vi "Control Experiment SM.vi"() -> ()   [LabVIEW 2016, in "Control Experiment SM.lvclass"]
doc: "Use this VI to help configure your experiment.\n1. Choose Pickering or Not Pickering\n2. Configure the Electrode control to show which electrode is connected to which lockin\n3. Choose a Label for each electrode to configure Krohn Hite amplifier automatically\n4. Easily set all Krohn Hite channels to be \"all ground\" or \"all differential\" mode\n5. Fill out information about you and your device in the lower left corner\n6. When you are finished, or when you want to update the amplifiers, click the \"CREATE OUTPUT\" button located in upper right. Clicking this button will set the amplifiers, Pickering switch (if you have one), and write information to a functional global variable that you can easily read from elsewhere in your program"
uses:
  Control Experiment SM.lvclass
  <vilib>/addons/_JKI.lib/Serialization/JSON/JKI JSON Serialization.lvlib
  Typedefs/KH Mode-enum.ctl
  <userlib>/LevyLab/Krohn Hite 7008/typedefs/Gain-Enum.ctl
  <userlib>/LevyLab/Krohn Hite 7008/Instrument.KH7008.lvclass
  <userlib>/LevyLab/Krohn Hite 7008/typedefs/Shunt-Enum.ctl
  <userlib>/LevyLab/Krohn Hite 7008/typedefs/Input Configuration-Enum.ctl
  <userlib>/_MGI/File/MGI Create Directory Chain Behavior Enum.ctl
  <vilib>/addons/_JKI.lib/REST Client/classes/REST Client/HTTP Header.ctl
  <vilib>/addons/_JKI.lib/REST Client/classes/REST Client/REST Client.lvclass
  <vilib>/JKI/JKI SMO/SMO/SMO.lvclass
  <userlib>/LevyLab/Lockin-Multichannel/Instrument.Lockin/Instrument.Lockin.lvclass
  Typedefs/Control Experiment JSON--cluster.ctl
  <vilib>/Utility/sysdir.llb/System Directory Type.ctl
  <userlib>/LevyLab/Levylab Instruments/SMOs/Configuration/Configuration.lvclass
  Typedefs/Instrument--enum.ctl
  Typedefs/UI Controls --cluster.ctl
  <userlib>/_OpenG.lib/array/array.llb/Remove Duplicates from 1D Array (Variant)__ogtk.vi
  <userlib>/LevyLab/Krohn Hite 7008/typedefs/Channel-Enum.ctl
  <userlib>/LevyLab/Krohn Hite 7008/typedefs/Filter-Enum.ctl
  <userlib>/LevyLab/Krohn Hite 7008/typedefs/Coupling-Enum.ctl
  <userlib>/LevyLab/Krohn Hite 7008/typedefs/SetAll-Cluster.ctl
  <userlib>/LevyLab/Krohn Hite 7008/typedefs/SetAll-Array.ctl
  <userlib>/LevyLab/Levylab Instruments/SMOs/Logger.PGSQL/Logger.PGSQL.lvclass
  <userlib>/_OpenG.lib/file/file.llb/File Exists - Scalar__ogtk.vi
  <vilib>/Platform/browser.llb/Open URL in Default Browser (string).vi
  <userlib>/LevyLab/Levylab Instruments/Instrument Types/CBridge/Instrument.CBridge.lvclass
  <userlib>/LevyLab/Levylab Instruments/Instrument Types/Strain/Instrument.Strain.lvclass
  C:/Program Files (x86)/National Instruments/LabVIEW 2016/vi.lib/JKI/JKI SMO/SMO/SMO.lvclass
  <userlib>/LevyLab/Levylab Instruments/Instrument Types/Cryostat/Instrument.Cryostat.lvclass
  <userlib>/LevyLab/Levylab Instruments/Instrument Types/Optical Delay Line/Instrument.OpticalDelayLine.lvclass
  <userlib>/LevyLab/Levylab Instruments/Instrument Types/VNA/Instrument.VNA.lvclass
  <userlib>/LevyLab/Levylab Instruments/Instrument Types/VSource/Instrument.VSource.lvclass
panel:
  in  "I'm Finished Taking Data!":bool
  out "Values have changed":bool
  in  "Create Output":bool
  in  "OK":bool
  out "Control Experiment":refnum<class "Control Experiment SM.lvclass">
  in  "C.E.":refnum<class "Control Experiment SM.lvclass">
  in  "Tab Control":T1(tab)
  in  "DC Coupled":bool=TRUE
  in  "Bandwidth Filter":bool=TRUE
  in  "#AO":u32=8
  in  "Gain":dbl[](array[numeric])=[1.0, 1.0, 1.0, 1.0, 1.0, 1.0, 1.0, 1.0]
  in  "KH":T5={"KH #"=[0, 1, 2, 3, 4, 5, 6, 7], "KH Configuration"=[enum."Differential", enum."Differential", enum."SE+ (-gnd)", enum."SE+ (-gnd)", enum."Ground", enum."Differential", enum."Ground", enum."Differential"], "KH Gain"=[enum."1x", enum."1000x", enum."1x", enum."10x", enum."1x", enum."1x", enum."1x", enum."1x"], "KH Shunt Resistor"=[enum."50k Ohms", enum."50k Ohms", enum."Open", enum."Open", enum."Open", enum."50k Ohms", enum."Open", enum."Open"]}
  in  "Lockin":T7={"AI"=[1, 2, 3, 4, 5, 6, 7, 8], "Electrode"=["1", "2", "4", "3", "", "26", "", ""], "Label"=[2, 14, 3, 4, 0, 1, 0, 0], "Electrode Config"=[enum."Current", enum."Gate", enum."Voltage (SE)", enum."Voltage (SE)", enum."Ground", enum."Current", enum."Ground", enum."Voltage (Diff)"]} {"Label" items=["", "I+", "I-", "V1+", "V1-", "V2+", "V2-", "V3+", "V3-", "V4+", "V4-", "dV1", "dV2", "dV3", "Vsg", "Vbg"]}
  in  "#AI":u32=8
  in  "KH All Buttons":T8(radio)
  in  "Defualt Shunt Resistor":T4=enum."50k Ohms"
  in  "Description":string="this is a test"
  in  "Sample (SAXXXX)":string="TEST"
  in  "Device (YYYYMMDD)":string="20200113"
  in  "Instrument":T9
  in  "Username":string="Patrick"
  in  "non KH":T10={"AO"=[], "Electrodes 2"=["27"], "Labels 2"=[1], "unused"=[]} {"Labels 2" items=["", "I+", "I-", "V1+", "V1-", "V2+", "V2-", "V3+", "V3-", "V4+", "V4-", "dV1", "dV2", "dV3", "Vsg", "Vbg"]}
  in  "Strain Cell Address":refnum<visa-resource-name>="GPIB0::INSTR38"
  in  "Capacitance Bridge Address":refnum<visa-resource-name>
  in  "C Bridge?":bool=TRUE
  in  "Strain Cell?":bool=TRUE
  in  "Pickering?":bool
  in  "Krohn Hite?":bool=TRUE
  in  "KH Addresses":refnum<visa-resource-name>[](array[refnum])=["COM1"] caption="KH Address[A,B,C,...]"
  in  "Lockin Address":string
  in  "Ring":u16(ring) items=["----Sweep Control----", "Sweep Control.vi", "Continuous B Sweep.vi", "----Transport----", "IV.vi", "IV_Sweep.vi", "Lockin_time.vi", "Lockin_Vsg.vi", "Lockin_sweep.vi", "Lockin_AIWFM_time.vi", "THz_TimeDelay.vi", "Sweep_AIWFM_time.vi"]
  in  "Open VI":bool
  in  "Open Lockin":bool
  in  "Pickering Enum":T11(ring)=enum."Pickering 4 Wire PPMS DR"
  in  "Write Pickering Config":bool
  in  "Read Pickering Config":bool
  in  "X Channels":string[](array[combo])=["x1", "x2", "x3", "x4", "x5", "x6", "x7", "x8", "x9", "x10", "x11", "x12"]
  in  "Electrodes (Pickering)":T12(array[ring])
  in  "Y Channels":string[][](array[combo])=[["y1", "NC"], ["y2", "NC"], ["y3", ""], ["y4", ""], ["y5", ""], ["y6", ""], ["y7", ""], ["y8", ""], ["NC", ""], ["y7", ""], ["y6", ""]]
  in  "Labels (Pickering)":u16[](array[ring]) items=["", "I+", "I-", "V1+", "V1-", "V2+", "V2-", "V3+", "V3-", "V4+", "V4-", "Vsg", "Vbg"]
  out "Y Channel Array":string[][](array[string])
  out "X Channel Array":string[](array[string])
  in  "AWS Credentials":path=path "G:/My Drive/ansom/Data" caption="AWS Credentials (File with AWS access key and secret access key"
  out "Refresh Token Out":string="0/0ccae0b202a2d5ce21e5be9cd72246b8"
  in  "Default Path":path=path "G:/My Drive/ansom/Data" caption="Default Path (Do not add your instrument name here)(Typ. G:\\My Drive\\ansom\\Data)"
  out "Comments":string="Device: \r  Device Name: TEST.20200113\r  Computer: ASTARTES\r  User: Patrick\r  Instrument: AGILENT\r  Description: |\r    this is a test\r\rExperiment: \r  Time: 2020-02-25T09:02:18\r  Description: |\r\rSweep: \r- Loop1: [OFF, 0.000000]\r- Loop2: [OFF, 0.000000]\r- Loop3: [OFF, 0.000000]\r- Loop4: [OFF, 0.000000]\r\rWiring: \r- Electrode 27: Lockin 1, I+, KH1 Channel 1, Differential, 1x, 50k Ohms\r\rLockin: \r  AO: \r  \r  REF: \r  \r  Sampling: \r  - Fs: \r  - N: \r"
  out "Device Folder":path=path "G:/My Drive/ansom/Data/AGILENT/TEST.20200113" caption="(\\base path\\project\\device\\ )"
  out "JSON String":string="{\r\n    \"Device\":{\r\n        \"Device\":\"TEST.20200113\",\r\n        \"User\":\"Patrick\",\r\n        \"Time\":\"2020-02-25T09:02:24\",\r\n        \"Computer Name\":\"ASTARTES\"\r\n    },\r\n    \"Wiring\":{\r\n        \"Lockin Ch\":[\r\n            1,\r\n            2,\r\n            3,\r\n            4,\r\n            5,\r\n            6,\r\n            7,\r\n            8\r\n        ],\r\n        \"KH Electrodes\":[\r\n            \"27\"\r\n        ],\r\n        \"KH Labels\":[\r\n            \"I+\"\r\n        ],\r\n        \"Other Electrodes\":[\r\n            \"27\"\r\n        ],\r\n        \"Other Labels\":[\r\n            \"I+\"\r\n        ]\r\n    }\r\n}"
  in  "Labels Strings":string[](array[string])=["", "I+", "I-", "V1+", "V1-", "V2+", "V2-", "V3+", "V3-", "V4+", "V4-", "dV1", "dV2", "dV3", "Vsg", "Vbg"]
  out "YAML example":string="description: This is a dummy dataset which mimics smFRET data.\n\nsetup:\n    ## Mandatory fields\n    num_pixels: 2                # using 2 detectors\n    num_spots: 1                 # a single confocal excitation\n    num_spectral_ch: 2           # donor and acceptor detection\n    num_polarization_ch: 1       # no polarization selection\n    num_split_ch: 1              # no beam splitter\n    modulated_excitation: False  # CW excitation, no modulation\n    lifetime: False              # no TCSPC in detection\n\n    ## Optional fields\n    excitation_wavelengths:      # List of excitation wavelenghts\n       - !!float 532e-9\n    excitation_cw:               # List of booleans, True if wavelength is CW\n       - True\n    detection_wavelengths:       # Nominal center wavelength for each for detection ch\n       - !!float 580e-9\n       - !!float 640e-9\n\nsample:\n  sample_name: describe the sample here\n  buffer_name: describe the buffer here\n  dye_names: 'Cy3B, ATTO647N'   # Comma separates names of fluorophores\n\nidentity:\n    author: Author Name\n    author_affiliation: Name of Research Institution\n\nprovenance:\n    filename: 'photon_data.hdf5'\n    software: Acquisition Software Name\n\nphoton_data:\n    timestamps_specs:\n        timestamps_unit: !!float 10e-9  # 10 ns\n    measurement_specs:\n        measurement_type: smFRET\n        detectors_specs:\n            spectral_ch1: [0]  # list of donor's detector IDs\n            spectral_ch2: [1]  # list of acceptor's detector IDs"
  in  "String":string
  # "SANDBOX:"
  # "Sample"
  # "Krohn Hite"
  # "Lockin"
  # "Lockin"
  # "Krohn Hite"
  # "Other"
  # "Device and Project Description"
  # "Hardware Configuration"
  # "Experiment VIs"
  # "Lockin (Local)"
  # "Path Configuration"
  # "Use this VI to help configure your experiment.\n1. Choose Pickering or Not Pickering\n2. Configure the Electrode control to show which electrode is connected to which lockin\n3. Choose a Label for each electrode to configure Krohn Hite amplifier automatically\n4. Easily set all Krohn Hite channels to be \"all ground\" or \"all differential\" mode\n5. Fill out information about you and your device in the lower left corner\n6. When you are finished, or when you want to update the amplifiers, click the \"CREATE OUTPUT\" button located in upper right.\nClicking this button will set the amplifiers, Pickering switch (if you have one), and write information to a functional global variable that you can easily read from elsewhere in your program"
  # "If you want to have new labels for the \"Labels\" field you can type them here"
  # "The magic words are:\nI\nVsg\nVbg\ndV\nV"
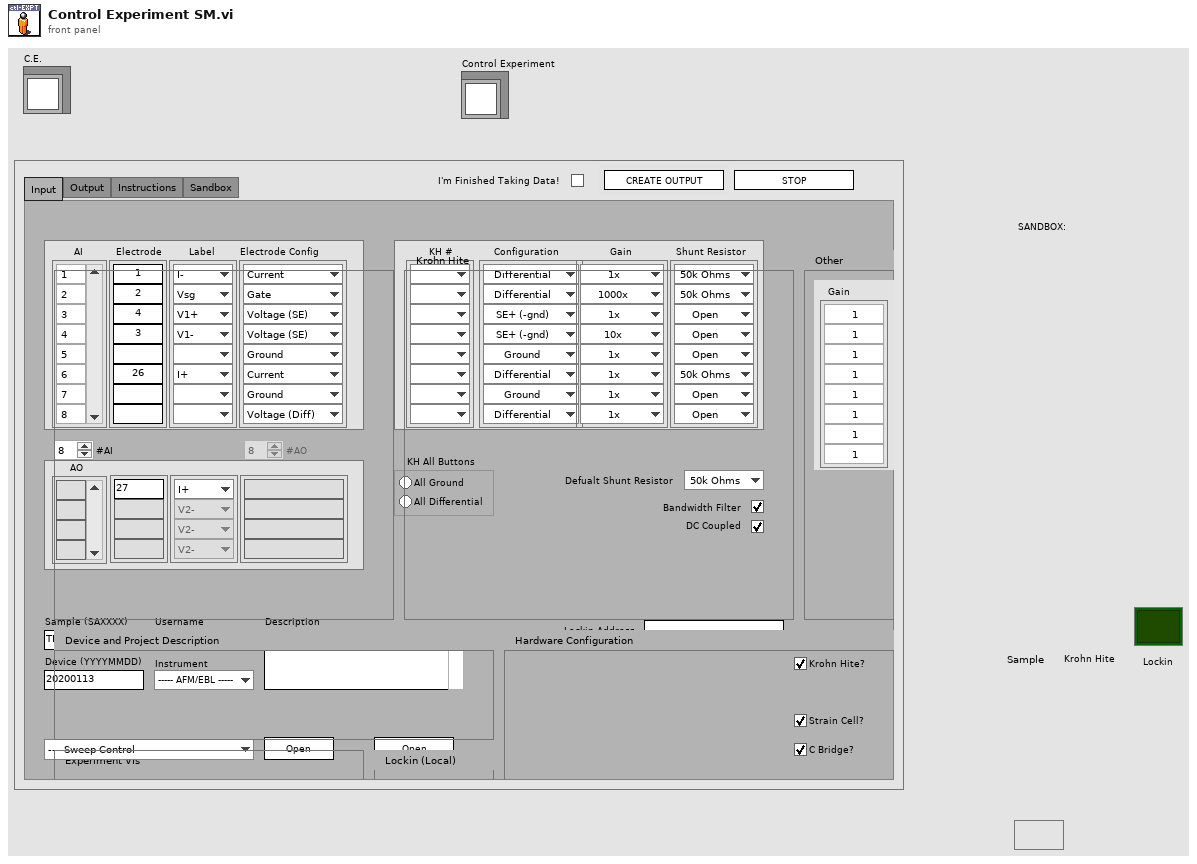
[diagram p1: front panel]
types:
  T1 = enum32{"Input", "Pickering", "Output", "Instructions", "Sandbox"}
  T2 = typedef "Instrument.KH7008.lvclass/Input Configuration-Enum.ctl" = enum16{"Ground", "SE+ (-gnd)", "SE- (+gnd)", "Differential"}
  T3 = typedef "Instrument.KH7008.lvclass/Gain-Enum.ctl" = enum16{"1x", "10x", "100x", "1000x"}
  T4 = typedef "Instrument.KH7008.lvclass/Shunt-Enum.ctl" = enum16{"Open", "50 Ohms", "500 Ohms", "5k Ohms", "50k Ohms", "10M Ohm"}
  T5 = cluster{"KH #":u16[], "KH Configuration":T2[], "KH Gain":T3[], "KH Shunt Resistor":T4[]}
  T6 = typedef "Control Experiment SM.lvclass/KH Mode-enum.ctl" = enum16{"Ground", "Current", "Voltage (SE)", "Voltage (Diff)", "Gate"}
  T7 = cluster{"AI":u32[], "Electrode":string[], "Label":u16[], "Electrode Config":T6[]}
  T8 = enum32{"No Selection", "All Ground", "All Differential"}
  T9 = typedef "Control Experiment SM.lvclass/Instrument--enum.ctl" = enum16{"----- AFM/EBL -----", "AGILENT", "CYPHER", "Gemini2", "JEOL", "MFP3D", "----- Cryostat -----", "CF900", "DR200", "MNK", "PPMS 1", "PPMS 2", "PPMS 3", "----- Optics -----", "THz 1", "THz 2"}
  T10 = cluster{"AO":string[], "Electrodes 2":string[], "Labels 2":u16[], "unused":string[]}
  T11 = enum16{"Pickering 4 Wire", "Pickering 4 Wire PPMS DR"}
  T12 = enum16{"NC", "26", "27", "28", "1", "2", "3", "4", "5", "6", "7", "8", "9", "10", "11", "12", "13", "14", "15", "16", "17", "18", "19", "20", "21", "22", "23", "24", "25"}[]
  T13 = enum16{"A 1", "A 2", "A 3", "A 4", "A 5", "A 6", "A 7", "A 8", "B 1", "B 2", "B 3", "B 4", "B 5", "B 6", "B 7", "B 8", "none"}
  T14 = enum8{"Enabled", "Disabled", "Disabled and Grayed Out"}
  T15 = enum32{"invalid app kind", "Development System", "Run Time System", "Student Edition", "Embedded LabVIEW", "Evaluation", "Custom"}
  T16 = enum32{"Invalid", "Standard", "Closed", "Hidden", "Minimized", "Maximized"}
  T17 = typedef "MGI Create Directory Chain Behavior Enum.ctl" = enum16{"Auto Detect", "Path Contains a File", "Path Does Not Contain a File"}
  T18 = typedef "Instrument.KH7008.lvclass/SetAll-Cluster.ctl" = cluster{"Channel":T19, "Gain":T3, "Bandwidth Filter":T20, "Shunt Resistor":T4, "Coupling":T21, "Input Config":T2}
  T19 = typedef "Instrument.KH7008.lvclass/Channel-Enum.ctl" = enum16{"Channel 1", "Channel 2", "Channel 3", "Channel 4", "Channel 5", "Channel 6", "Channel 7", "Channel 8"}
  T20 = typedef "Instrument.KH7008.lvclass/Filter-Enum.ctl" = enum16{"OFF", "ON"}
  T21 = typedef "Instrument.KH7008.lvclass/Coupling-Enum.ctl" = enum16{"AC", "DC"}
  T22 = enum16{"GSR", "Research Projects", "Undergrads", "Researchers", "Hardware", "Software", "LevyLab", "Samples", "Manuscripts", "AoT", "WorkStudy"}
  T23 = cluster{"26":string[], "27":string[], "28":string[], "1":string[], "2":string[], "3":string[], "4":string[], "5":string[]}
  T24 = enum16{"A 1", "A 2", "A 3", "A 4", "A 5", "A 6", "A 7", "A 8", "B 1", "B 2", "B 3", "B 4", "B 5", "B 6", "B 7", "B 8", "none"}[]
  T25 = typedef "Control Experiment SM.lvclass/Experiment Description--cluster.ctl" = cluster{"User":string, "Device":string, "Device Path":path, "Device Description":string, "Experiment Path":path, "Experiment Description":string, "Instrument":T9, "Sweep":cluster{"key":string, "value":variant}[], "Device Description JSON":string, "Experiment Description JSON":string}
  T26 = typedef "Control Experiment SM.lvclass/Wiring Description--cluster.ctl" = cluster{"Lockin Ch":i32[], "KH":cluster{"Electrodes":string[], "Labels":string[]}, "not KH":cluster{"Electrodes":string[], "Labels":string[]}}
  T27 = typedef "Instrument.KH7008.lvclass/SetAll-Array.ctl" = T18[]
  T28 = typedef "Control Experiment SM.lvclass/UI Controls --cluster.ctl" = cluster{"Sample":string, "Device":string, "Username":string, "Description":string, "Default Path":path, "AWS Path":path, "Instrument":T9, "Lockin?":bool, "Lockin Address":string, "Krohn Hite?":bool, "KH Addresses":refnum<visa-resource-name>[], "KH All Buttons":enum32{"No Selection", "All Ground", "All Differential"}, "Strain Cell?":bool, "Strain Cell Address":refnum<visa-resource-name>, "C Bridge?":bool, "Capacitance Bridge Address":refnum<visa-resource-name>, "Lockin":cluster{"AI":u32[], "Electrode":string[], "Label":u16[], "Electrode Config":T6[]}, "KH":cluster{"KH #":enum16{"A 1", "A 2", "A 3", "A 4", "A 5", "A 6", "A 7", "A 8", "B 1", "B 2", "B 3", "B 4", "B 5", "B 6", "B 7", "B 8", "none"}[], "KH Configuration":T2[], "KH Gain":T3[], "KH Shunt Resistor":T4[], "Filter":bool, "DC Coupled":bool}, "non KH":cluster{"Scroll Bar":string[], "Electrodes 2":string[], "Labels 2":u16[], "unused":string[]}, "#AI":u32}
  T29 = typedef "REST Client.lvlib/REST Client.lvclass/HTTP Header.ctl" = cluster{"header":string, "value":string}
  T30 = cluster{"Core":cluster{"Current VI Reference":refnum<vi>, "Close Panel on Exit?":bool}, "C.E.":refnum<class "Control Experiment SM.lvclass">, "Experiment":T25, "Wiring Configuration":T26, "Channel Settings":cluster{"Channel Setting":T27}[], "KH All Buttons":enum32{"No Selection", "All Ground", "All Differential"}, "Lockin":cluster{"AI":u32[], "Electrode":string[], "Label":u16[], "Electrode Config":T6[]}, "KH":cluster{"KH #":u16[], "KH Configuration":T2[], "KH Gain":T3[], "KH Shunt Resistor":T4[]}, "non KH":cluster{"AO":string[], "Electrodes 2":string[], "Labels 2":u16[], "unused":string[]}, "UI":T28, "Asana":cluster{"Authentication Info":cluster{"Client ID":string, "Client Secret":string, "Redirect URI":string, "Token Endpoint":string, "Scope":string}, "Authentication Header":T29[], "Refresh Token":string, "Time Stamp":timestamp}, "Logger":refnum<class "Logger.PGSQL.lvclass">, "Config":refnum<class "Configuration.lvclass">, "VI paths":path[]}
  T31 = cluster{"Authentication Info":cluster{"Client ID":string, "Client Secret":string, "Redirect URI":string, "Token Endpoint":string, "Scope":string}, "Authentication Header":T29[], "Refresh Token":string, "Time Stamp":timestamp}
  T32 = cluster{"Current VI Reference":refnum<vi>, "Close Panel on Exit?":bool}
  T33 = typedef "System Directory Type.ctl" = i32
  T34 = cluster{"Scroll Bar":string[], "Electrodes 2":string[], "Labels 2":u16[], "unused":string[]}
  T35 = typedef "Control Experiment SM.lvclass/Control Experiment JSON--cluster.ctl" = cluster{"Device":cluster{"Device":string, "User":string, "Time":string, "Computer Name":string}, "Wiring":cluster{"Lockin Ch":u32[], "KH Electrodes":string[], "KH Labels":string[], "Other Electrodes":string[], "Other Labels":string[]}}
  T36 = cluster{"Client ID":string, "Client Secret":string, "Redirect URI":string, "Token Endpoint":string, "Scope":string}
  T37 = cluster{"gid":string, "name":string, "resource_type":string}[]
  T38 = cluster{"id":i64, "gid":string, "resource_type":string, "name":string}[]
  T39 = cluster{"Electrodes (Pickering)":enum16{"NC", "26", "27", "28", "1", "2", "3", "4", "5", "6", "7", "8", "9", "10", "11", "12", "13", "14", "15", "16", "17", "18", "19", "20", "21", "22", "23", "24", "25"}[], "X Channels":string[]}
  T40 = cluster{"Labels (Pickering)":u16[], "Y Channels":string[][]}
  T41 = cluster{cluster{"Electrodes (Pickering)":enum16{"NC", "26", "27", "28", "1", "2", "3", "4", "5", "6", "7", "8", "9", "10", "11", "12", "13", "14", "15", "16", "17", "18", "19", "20", "21", "22", "23", "24", "25"}[], "X Channels":string[]}, cluster{"Labels (Pickering)":u16[], "Y Channels":string[][]}}
  T42 = cluster{"x config":cluster{"Electrode":enum16{"NC", "26", "27", "28", "1", "2", "3", "4", "5", "6", "7", "8", "9", "10", "11", "12", "13", "14", "15", "16", "17", "18", "19", "20", "21", "22", "23", "24", "25"}[], "X Channels":string[]}, "y config":cluster{"Label":u16[], "Y Channels":string[][]}}
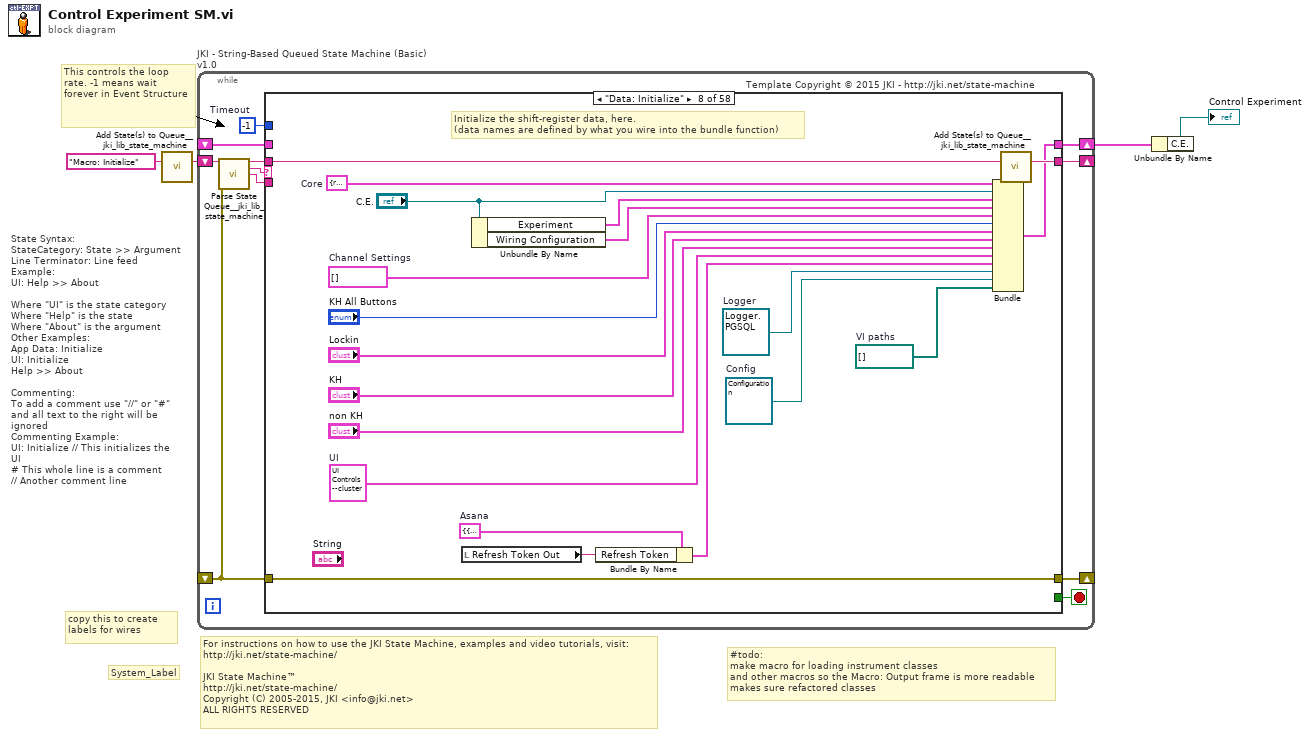
[diagram p0: block diagram]
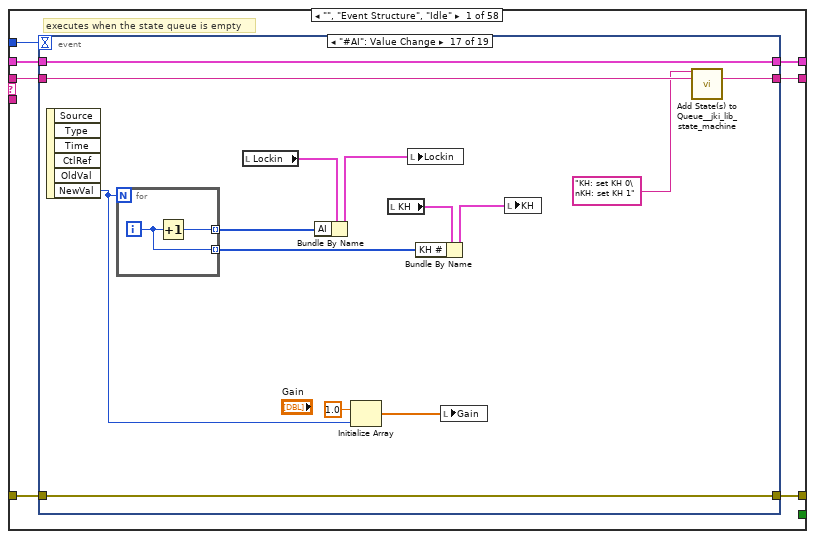
[diagram p2: hidden frame]
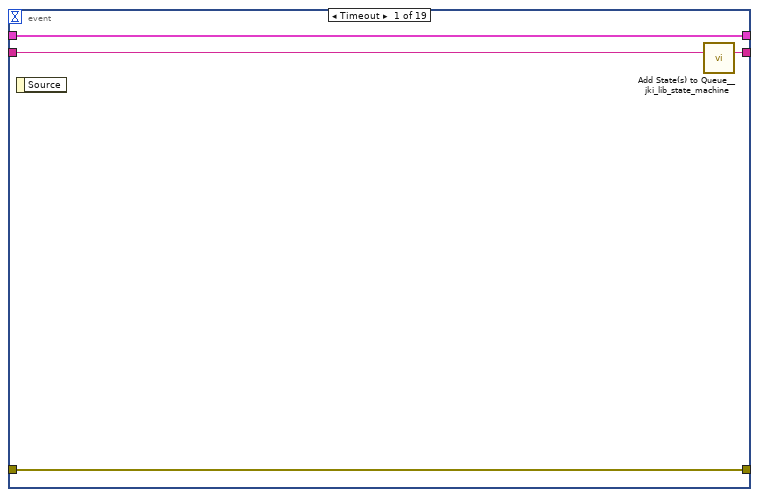
[diagram p3: hidden frame]
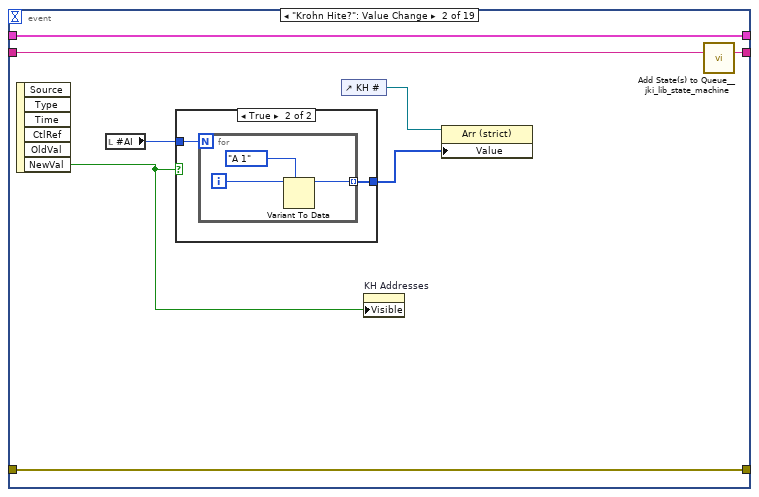
[diagram p4: hidden frame]
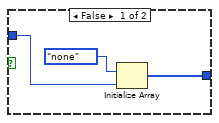
[diagram p5: hidden frame]
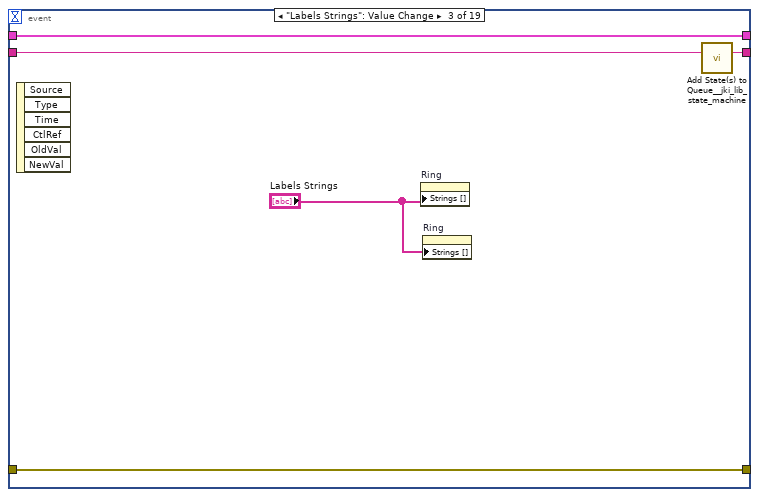
[diagram p6: hidden frame]
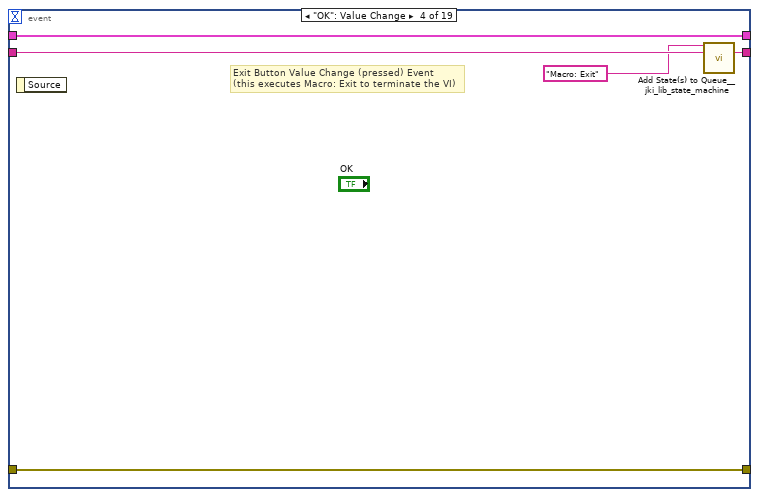
[diagram p7: hidden frame]
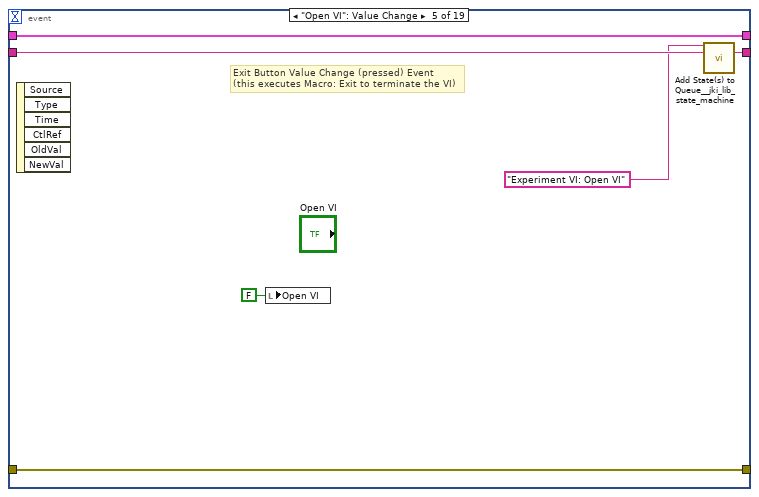
[diagram p8: hidden frame]
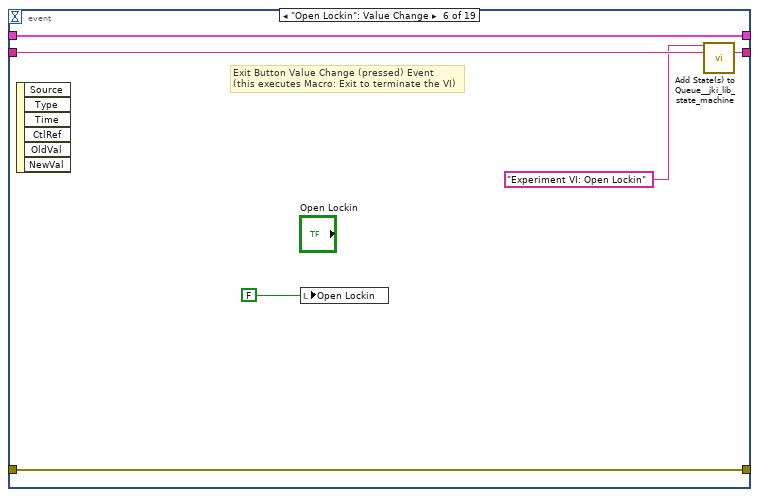
[diagram p9: hidden frame]
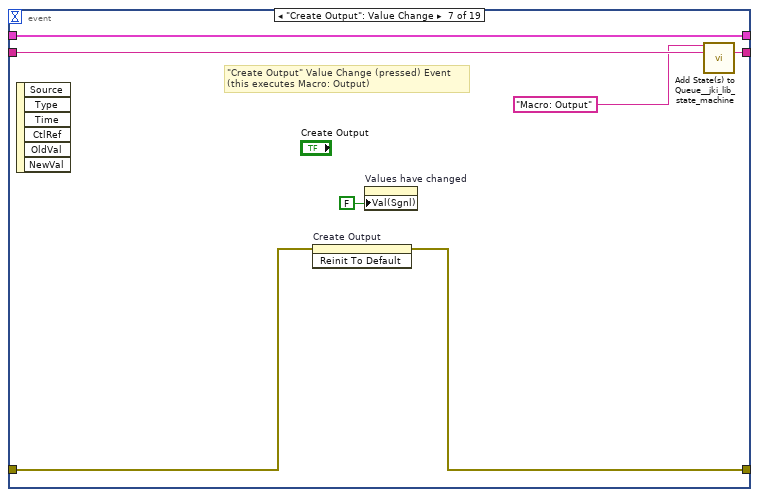
[diagram p10: hidden frame]
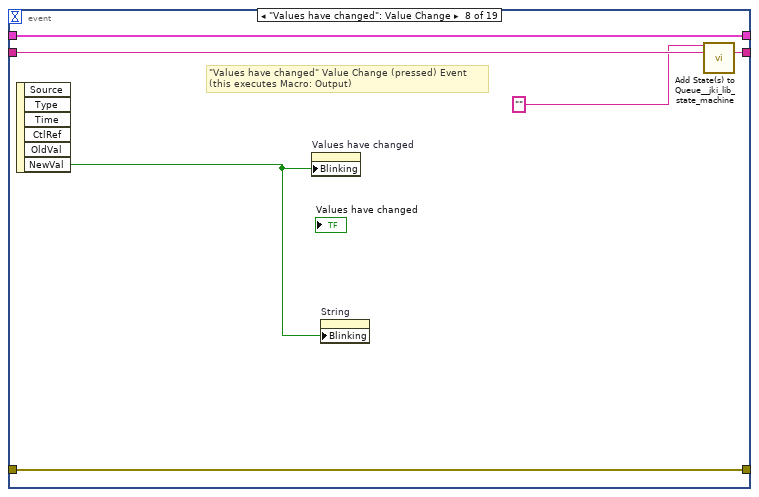
[diagram p11: hidden frame]
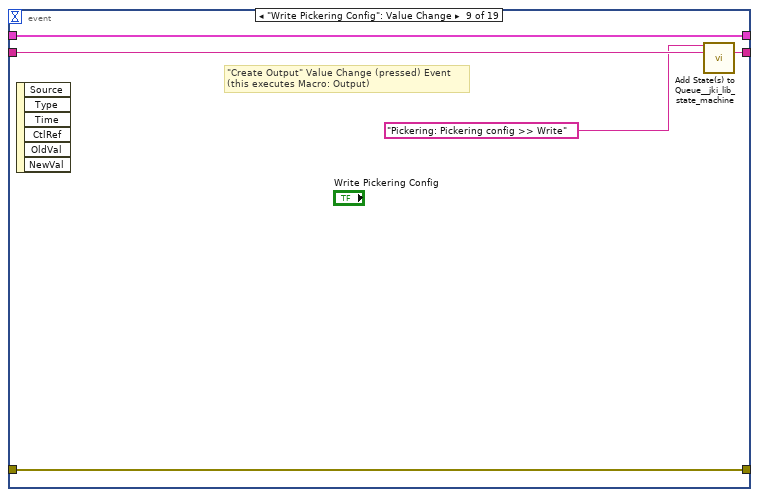
[diagram p12: hidden frame]
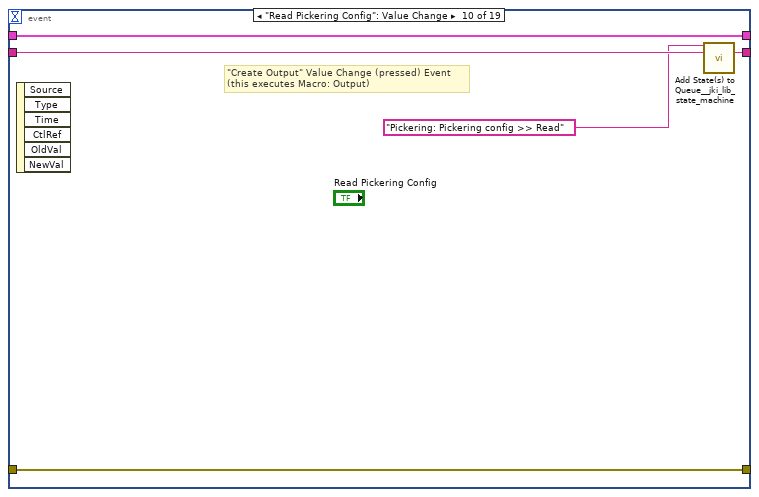
[diagram p13: hidden frame]
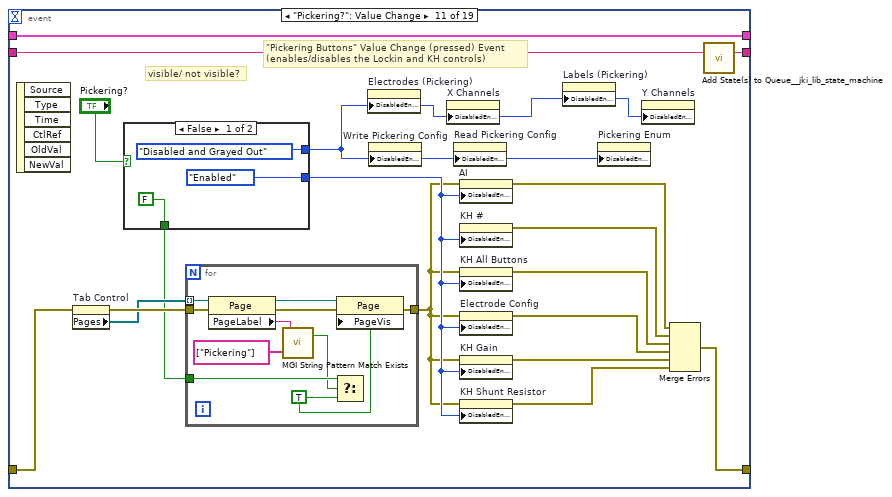
[diagram p14: hidden frame]
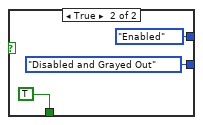
[diagram p15: hidden frame]
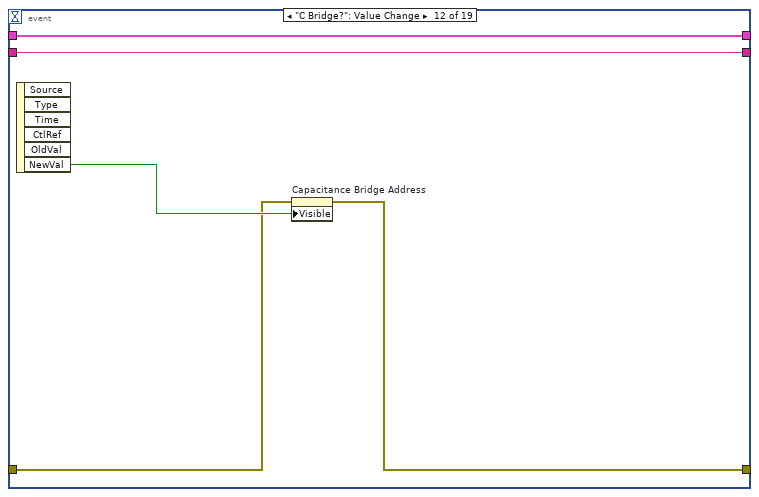
[diagram p16: hidden frame]
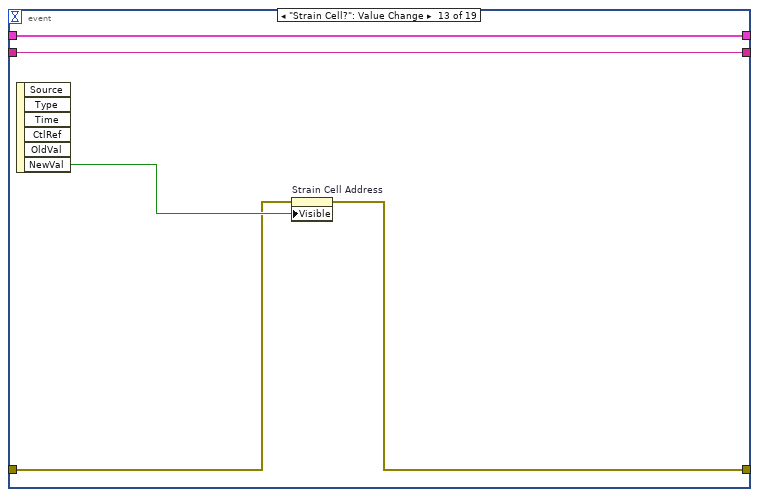
[diagram p17: hidden frame]
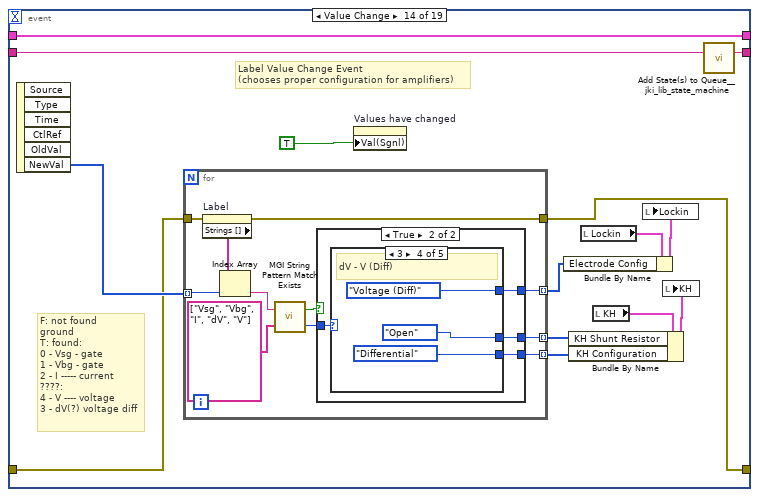
[diagram p18: hidden frame]
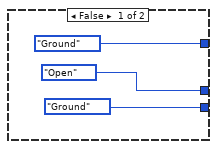
[diagram p19: hidden frame]
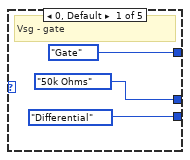
[diagram p20: hidden frame]
diagram:
  # "#todo:\nmake macro for loading instrument classes\nand other macros so the Macro: Output frame is more readable\nmakes sure refactored classes"
  # "For instructions on how to use the JKI State Machine, examples and video tutorials, visit:\nhttp://jki.net/state-machine/\n\nJKI State Machine™\nhttp://jki.net/state-machine/\nCopyright (C) 2005-2015, JKI <info@jki.net>\nALL RIGHTS RESERVED"
  # "State Syntax:\nStateCategory: State >> Argument\nLine Terminator: Line feed\nExample:\nUI: Help >> About\n\nWhere \"UI\" is the state category\nWhere \"Help\" is the state\nWhere \"About\" is the argument\nOther Examples:\nApp Data: Initialize\nUI: Initialize\nHelp >> About\n\nCommenting:\nTo add a comment use \"//\" or \"#\" and all text to the right will be ignored\nCommenting Example:\nUI: Initialize // This initializes the UI\n# This whole line is a comment\n// Another comment line"
  # "copy this to create labels for wires"
  # "This controls the loop rate. -1 means wait forever in Event Structure"
  # "System_Label"
  n1 = call <vilib>:"Add State(s) to Queue__jki_lib_state_machine.vi"("State(s) in (\"\")"="Macro: Initialize") -> ("States Out"=w4:string)  [unwired: 14 in]
  n2 = while "JKI - String-Based Queued State Machine (Basic) v1.0" {
    shift-right: [w8] -> w2
    shift-left: _ -> [w7]
    shift-right: [w11] -> _
    shift-left: _ -> [w5]
    shift-right: [w10] -> _
    shift-left: w4 -> [w12]
    stop <- w9 stop-if-true
    w6 = -1  # Timeout
    # "Template Copyright © 2015 JKI - http://jki.net/state-machine"
    n3 = call <vilib>:"Parse State Queue__jki_lib_state_machine.vi"("State Queue"=w12, "Error In (no error)"=w5) -> ("Remaining States"=w14:string, "Current State"=w15:string, "Arguments"=w13:string)  [unwired: 11 in]
    n4 = case shown="\"Data: Initialize\"" w15 {
      selector: w15 -> [_ _ w223 _ _ _ _ _ _ _ _ _ _ _ _ _ _ _ _ _ _ _ _ _ _ _ _ _ _ _ _ _ _ _ _ _ _ _ _ _ _ _ _ _ _ _ _ _ _ _ _ _ _ _ _ _ _ _]
      tunnel: w14 -> [w22 w222 w227 w245 w251 w256 w260 w280 w300 w338 w346 w350 w370 w404 w410 w421 w447 w462 w475 w479 w484 w495 w502 w518 w523 w528 w532 w544 w560 w586 w600 w616 w633 w640 w671 w675 w693 w726 w813 w828 w836 w847 w864 w879 w883 w891 w909 w940 w956 w977 w991 w996 w1000 w1010 w1028 w1032 w1039 w1070]
      tunnel: w13 -> [_ _ _ _ _ _ _ _ _ _ _ _ _ _ w405 w415 _ _ _ _ _ _ _ _ _ _ _ _ _ _ _ _ _ _ _ _ _ _ _ _ _ _ _ _ _ _ _ _ _ _ _ _ _ _ _ _ w1037 _]
      tunnel: w7 -> [w20 w219 w225 w236 w248 w254 w257 _ w296 w317 w341 w347 w358 w377 w408 w417 w444 w459 w473 w476 w481 w492 w500 w515 w520 w525 w529 w540 w556 w583 w598 w612 w631 w638 w643 w672 w691 w718 w804 w825 w834 w840 w860 w871 w880 w885 w893 w925 w953 w964 w989 w994 w997 w1002 w1026 w1029 w1034 w1060]
      tunnel: [w19 w220 w229 w242 errorcluster {"status"=FALSE, "code"=0, "source"=""} ("error out") w253 w258 w277 w291 w318 w344 w348 w359 w402 w406 w418 w445 w460 w463 w477 w482 w493 w498 w516 w521 w526 w530 w542 w558 w570 w591 w609 w621 w636 w644 w673 w677 w717 w810 w826 w830 w844 w858 w865 w881 w889 w902 w922 w954 w975 w984 w992 w998 w1003 w1014 w1030 w1036 w1066] -> w11
      tunnel: w5 -> [w18 w220 w228 w242 w247 w253 w258 w277 w297 w319 w342 w348 w368 w402 w407 w419 w445 w460 w470 w477 w482 w493 w498 w516 w521 w526 w530 w542 w558 w573 w592 w609 w622 w634 w659 w673 w687 w717 w799 w826 w829 w845 w861 w872 w881 w889 w892 w938 w954 w975 w985 w993 w998 w1004 w1016 w1030 w1035 w1064]
      tunnel: [w21 w221 w226 w244 w250 w255 w259 w279 w299 w337 w345 w349 w369 w403 w409 w420 w446 w461 w474 w478 w483 w494 w501 w517 w522 w527 w531 w543 w559 w585 w599 w615 w632 w639 w670 w674 w692 w725 w812 w827 w835 w846 w863 w878 w882 w890 w908 w939 w955 w976 w990 w995 w999 w1009 w1027 w1031 w1038 w1069] -> w10
      tunnel: [_ _ _ _ _ TRUE _ _ _ _ _ _ _ _ _ _ _ _ _ _ _ _ _ _ _ _ _ _ _ _ _ _ _ _ _ _ _ _ _ _ _ _ _ _ _ _ _ _ _ _ _ _ _ _ _ _ _ _] -> w9
      tunnel: [w17 w219 w225 w243 w248 w254 w257 w278 w295 w308 w341 w347 w358 w377 w408 w417 w444 w459 w473 w476 w481 w492 w500 w515 w520 w525 w529 w541 w557 w584 w597 w611 w630 w638 w642 w672 w690 w724 w811 w825 w833 w839 w859 w877 w880 w884 w903 w925 w953 w963 w989 w994 w997 w1001 w1026 w1029 w1034 w1060] -> w8
      tunnel: w6 -> [w16 _ _ _ _ _ _ _ _ _ _ _ _ _ _ _ _ _ _ _ _ _ _ _ _ _ _ _ _ _ _ _ _ _ _ _ _ _ _ _ _ _ _ _ _ _ _ _ _ _ _ _ _ _ _ _ _ _]
      frame "", "Event Structure", "Idle" {
        # "executes when the state queue is empty"
        n5 = event shown="[16] \"#AI\": Value Change" {
          selector: _ -> [_ _ _ _ _ _ _ _ _ _ _ _ _ _ _ _ _ _ _]
          dyn-events: _ -> [_ _ _ _ _ _ _ _ _ _ _ _ _ _ _ _ _ _ _]
          timeout: w16 -> [_ _ _ _ _ _ _ _ _ _ _ _ _ _ _ _ _ _ _]
          tunnel: w22 -> [w26 w34 w45 w52 w58 w64 w71 w77 w82 w87 w105 w123 w128 w145 w180 w185 w200 w212 w218]
          tunnel: [w25 w33 w47 w51 w57 w63 w70 w76 w81 w86 w104 w123 w128 w144 w180 w184 w199 w211 w217] -> w21
          tunnel: w20 -> [w23 w31 w46 w49 w55 w61 w69 w75 w80 w85 w103 w122 w127 w143 w181 w186 w198 w209 w215]
          tunnel: [w24 w32 w44 w50 w56 w62 w66 w73 w78 w83 w95 w124 w129 w132 w182 w187 w201 w210 w216] -> w19
          tunnel: w18 -> [w24 w32 w44 w50 w56 w62 w67 w73 w78 w83 w92 w125 w130 w141 w182 w187 w201 w210 w216]
          tunnel: [w23 w31 w46 w49 w55 w61 w69 w75 w80 w85 w103 w122 w127 w143 w181 w186 w198 w209 w215] -> w17
          event Timeout {
            n6 = event-data() -> ()  [unwired: 1 in, 1 out]
            n7 = call <vilib>:"Add State(s) to Queue__jki_lib_state_machine.vi"("State(s) in (\"\")"=w26) -> ("States Out"=w25:string)  [unwired: 14 in]
          }
          event "Krohn Hite?": Value Change {
            n8 = event-data() -> ("NewVal"=w27:bool)  [unwired: 1 in, 5 out]
            n9 = local read "#AI"() -> (w28:u32)
            n10 = case shown="True" w27 {
              tunnel: [w37 w38] -> w29
              tunnel: w28 -> [w36 w39]
              frame False {
                n11 = Initialize Array(T13."none" ("Enum"), w36) -> (w37:T24)
              }
              frame True {
                n12 = for {
                  N: w39 -> [_]
                  tunnel: [w40] -> w38 mode=indexing
                  i -> [w41]
                  n13 = Variant To Data(type=T13."A 1" ("Enum"), Variant=w41) -> (data=w40:T13)  [unwired: 1 in, 1 out]
                }
              }
            }
            n14 = control-ref of="KH #"() -> (w30:refnum<vi>)
            n15 = property on="KH Addresses" class="Arr (strict)"("Visible"=w27) -> ()  [unwired: 2 in, 2 out]
            n16 = property class="Arr (strict)"(reference=w30, "Value"=w29) -> ()  [unwired: 1 in, 2 out]
            n17 = call <vilib>:"Add State(s) to Queue__jki_lib_state_machine.vi"("State(s) in (\"\")"=w34) -> ("States Out"=w33:string)  [unwired: 14 in]
          }
          event "Labels Strings": Value Change {
            n18 = event-data() -> ()  [unwired: 1 in, 6 out]
            n19 = property on="Ring" class="Ring (strict)"("Strings []"="Labels Strings") -> ()  [unwired: 2 in, 2 out]
            n20 = property on="Ring" class="Ring (strict)"("Strings []"="Labels Strings") -> ()  [unwired: 2 in, 2 out]
            n21 = call <vilib>:"Add State(s) to Queue__jki_lib_state_machine.vi"("State(s) in (\"\")"=w45) -> ("States Out"=w47:string)  [unwired: 14 in]
          }
          event "OK": Value Change {
            # "Exit Button Value Change (pressed) Event\n(this executes Macro: Exit to terminate the VI)"
            n22 = event-data() -> ()  [unwired: 1 in, 1 out]
            n23 = call <vilib>:"Add State(s) to Queue__jki_lib_state_machine.vi"("State(s) in Front (\"\")"="Macro: Exit", "State(s) in (\"\")"=w52) -> ("States Out"=w51:string)  [unwired: 13 in]
          }
          event "Open VI": Value Change {
            # "Exit Button Value Change (pressed) Event\n(this executes Macro: Exit to terminate the VI)"
            n24 = event-data() -> ()  [unwired: 1 in, 6 out]
            n25 = local write "Open VI"(FALSE ("Open VI")) -> ()
            n26 = call <vilib>:"Add State(s) to Queue__jki_lib_state_machine.vi"("State(s) in Front (\"\")"="Experiment VI: Open VI", "State(s) in (\"\")"=w58) -> ("States Out"=w57:string)  [unwired: 13 in]
          }
          event "Open Lockin": Value Change {
            # "Exit Button Value Change (pressed) Event\n(this executes Macro: Exit to terminate the VI)"
            n27 = event-data() -> ()  [unwired: 1 in, 6 out]
            n28 = local write "Open Lockin"(FALSE ("Open VI")) -> ()
            n29 = call <vilib>:"Add State(s) to Queue__jki_lib_state_machine.vi"("State(s) in Front (\"\")"="Experiment VI: Open Lockin", "State(s) in (\"\")"=w64) -> ("States Out"=w63:string)  [unwired: 13 in]
          }
          event "Create Output": Value Change {
            # "\"Create Output\" Value Change (pressed) Event\n(this executes Macro: Output)"
            n30 = event-data() -> ()  [unwired: 1 in, 6 out]
            n31 = invoke on="Create Output" class="Bool" method="Reinit To Default"(error in=w67) -> (error out=w66:errorcluster)  [unwired: 2 in, 2 out]
            n32 = property on="Values have changed" class="Bool (strict)"("Val(Sgnl)"=FALSE ("Value (Signaling)")) -> ()  [unwired: 2 in, 2 out]
            n33 = call <vilib>:"Add State(s) to Queue__jki_lib_state_machine.vi"("State(s) in Front (\"\")"="Macro: Output", "State(s) in (\"\")"=w71) -> ("States Out"=w70:string)  [unwired: 13 in]
          }
          event "Values have changed": Value Change {
            # "\"Values have changed\" Value Change (pressed) Event\n(this executes Macro: Output)"
            n34 = event-data() -> ("NewVal"=w72:bool)  [unwired: 1 in, 5 out]
            n35 = property on="Values have changed" class="Bool (strict)"("Blinking"=w72) -> ()  [unwired: 2 in, 2 out]
            n36 = property on="String" class="Str"("Blinking"=w72) -> ()  [unwired: 2 in, 2 out]
            n37 = call <vilib>:"Add State(s) to Queue__jki_lib_state_machine.vi"("State(s) in Front (\"\")"="", "State(s) in (\"\")"=w77) -> ("States Out"=w76:string)  [unwired: 13 in]
          }
          event "Write Pickering Config": Value Change {
            # "\"Create Output\" Value Change (pressed) Event\n(this executes Macro: Output)"
            n38 = event-data() -> ()  [unwired: 1 in, 6 out]
            n39 = call <vilib>:"Add State(s) to Queue__jki_lib_state_machine.vi"("State(s) in Front (\"\")"="Pickering: Pickering config >> Write", "State(s) in (\"\")"=w82) -> ("States Out"=w81:string)  [unwired: 13 in]
          }
          event "Read Pickering Config": Value Change {
            # "\"Create Output\" Value Change (pressed) Event\n(this executes Macro: Output)"
            n40 = event-data() -> ()  [unwired: 1 in, 6 out]
            n41 = call <vilib>:"Add State(s) to Queue__jki_lib_state_machine.vi"("State(s) in Front (\"\")"="Pickering: Pickering config >> Read", "State(s) in (\"\")"=w87) -> ("States Out"=w86:string)  [unwired: 13 in]
          }
          event "Pickering?": Value Change {
            # "visible/ not visible?"
            # "\"Pickering Buttons\" Value Change (pressed) Event\n(enables/disables the Lockin and KH controls)"
            n42 = event-data() -> ()  [unwired: 1 in, 6 out]
            n43 = property on="Tab Control" class="TabCtl (strict)"(error in=w92) -> (error out=w94:errorcluster, "Pages"=w93:refnum<vi>[])  [unwired: 1 in, 1 out]
            n44 = case shown="False" "Pickering?" {
              tunnel: [T14."Enabled" ("Disabled") T14."Disabled and Grayed Out" ("Disabled")] -> w102
              tunnel: [FALSE ("Page Visible") TRUE ("Page Visible")] -> w89
              tunnel: [T14."Disabled and Grayed Out" ("Disabled") T14."Enabled" ("Disabled")] -> w88
              frame False {
              }
              frame True {
              }
            }
            n45 = for {
              tunnel: w93 -> [w115] mode=indexing
              tunnel: w94 -> [w111]
              tunnel: w89 -> [w108]
              tunnel: [w109] -> w91
              w106 = TRUE ("Page Visible")
              n46 = property class="Page"(reference=w115, error in=w111) -> (reference out=w112:refnum<vi>, error out=w110:errorcluster, "PageLabel"=w114:string)
              n47 = call <userlib>:"MGI String Pattern Match Exists.vi"("Patterns to Try"=string[] ["Pickering"], "String"=w114) -> ("Match Found"=w107:bool)  [unwired: 1 out]
              n48 = Select(t=w108, s=w107, f=w106) -> ()  [unwired: 1 out]
              n49 = property class="Page"(reference=w112, error in=w110, "PageVis"=w106) -> (error out=w109:errorcluster)  [unwired: 1 out]
            }
            n50 = property on="Electrodes (Pickering)" class="Arr (strict)"("DisabledEnum"=w88) -> ()  [unwired: 2 in, 2 out]
            n51 = property on="Write Pickering Config" class="Bool"("DisabledEnum"=w88) -> ()  [unwired: 2 in, 2 out]
            n52 = property on="X Channels" class="Arr (strict)"("DisabledEnum"=w88) -> ()  [unwired: 2 in, 2 out]
            n53 = property on="Read Pickering Config" class="Bool"("DisabledEnum"=w88) -> ()  [unwired: 2 in, 2 out]
            n54 = property on="AI" class="Arr (strict)"(error in=w91, "DisabledEnum"=w102) -> (error out=w96:errorcluster)  [unwired: 1 in, 1 out]
            n55 = property on="KH #" class="Arr (strict)"("DisabledEnum"=w102) -> (error out=w97:errorcluster)  [unwired: 2 in, 1 out]
            n56 = property on="KH All Buttons" class="RadioBtnsControl (strict)"(error in=w91, "DisabledEnum"=w102) -> (error out=w98:errorcluster)  [unwired: 1 in, 1 out]
            n57 = property on="Electrode Config" class="Arr (strict)"(error in=w91, "DisabledEnum"=w102) -> (error out=w99:errorcluster)  [unwired: 1 in, 1 out]
            n58 = property on="KH Gain" class="Arr (strict)"(error in=w91, "DisabledEnum"=w102) -> (error out=w100:errorcluster)  [unwired: 1 in, 1 out]
            n59 = property on="KH Shunt Resistor" class="Arr (strict)"(error in=w91, "DisabledEnum"=w102) -> (error out=w101:errorcluster)  [unwired: 1 in, 1 out]
            n60 = property on="Labels (Pickering)" class="Arr (strict)"("DisabledEnum"=w88) -> ()  [unwired: 2 in, 2 out]
            n61 = property on="Pickering Enum" class="Enum (strict)"("DisabledEnum"=w88) -> ()  [unwired: 2 in, 2 out]
            n62 = property on="Y Channels" class="Arr (strict)"("DisabledEnum"=w88) -> ()  [unwired: 2 in, 2 out]
            n63 = Merge Errors(w96, w97, w98, w99, w100, w101) -> (w95:errorcluster)
            n64 = call <vilib>:"Add State(s) to Queue__jki_lib_state_machine.vi"("State(s) in (\"\")"=w105) -> ("States Out"=w104:string)  [unwired: 14 in]
          }
          event "C Bridge?": Value Change {
            n65 = event-data() -> ("NewVal"=w126:bool)  [unwired: 1 in, 5 out]
            n66 = property on="Capacitance Bridge Address" class="VISAName"(error in=w125, "Visible"=w126) -> (error out=w124:errorcluster)  [unwired: 1 in, 1 out]
          }
          event "Strain Cell?": Value Change {
            n67 = event-data() -> ("NewVal"=w131:bool)  [unwired: 1 in, 5 out]
            n68 = property on="Strain Cell Address" class="VISAName"(error in=w130, "Visible"=w131) -> (error out=w129:errorcluster)  [unwired: 1 in, 1 out]
          }
          event "Lockin.Label": Value Change {
            # "F: not found\nground\nT: found:\n0 - Vsg - gate\n1 - Vbg - gate\n2 - I ----- current\n????:\n4 - V ---- voltage\n3 - dV(?) voltage diff"
            # "Label Value Change Event\n(chooses proper configuration for amplifiers)"
            n69 = event-data() -> ("NewVal"=w142:u16[])  [unwired: 1 in, 5 out]
            n70 = for {
              tunnel: w142 -> [w153] mode=indexing
              tunnel: [w155] -> w137 mode=indexing
              tunnel: w141 -> [w152]
              tunnel: [w151] -> w132
              tunnel: [w150] -> w134 mode=indexing
              tunnel: [w146] -> w135 mode=indexing
              n71 = property on="Label" class="Ring (strict)"(error in=w152) -> (error out=w151:errorcluster, "Strings []"=w154:string[])  [unwired: 1 in, 1 out]
              n72 = Index Array(array=w154, index=w153) -> (element=w149:string)
              n73 = call <userlib>:"MGI String Pattern Match Exists.vi"("Patterns to Try"=string[] ["Vsg", "Vbg", "I", "dV", "V"], "String"=w149) -> ("Index of First Pattern Matched"=w156:i32, "Match Found"=w147:bool)
              n74 = case shown="True" w147 {
                tunnel: w156 -> [_ w163]
                tunnel: [KH_Mode-enum."Ground" ("Enum") w162] -> w155
                tunnel: [Shunt-Enum."Open" ("Shunt Resistor") w161] -> w150
                tunnel: [Input_Configuration-Enum."Ground" ("Input Configuation") w160] -> w146
                frame False {
                }
                frame True {
                  n75 = case shown="3" w163 {
                    tunnel: [KH_Mode-enum."Gate" ("Enum") KH_Mode-enum."Gate" ("Enum") KH_Mode-enum."Current" ("Enum") KH_Mode-enum."Voltage (Diff)" ("Enum") KH_Mode-enum."Voltage (SE)" ("Enum")] -> w162
                    tunnel: [Shunt-Enum."50k Ohms" ("Shunt Resistor") Shunt-Enum."50k Ohms" ("Shunt Resistor") "Defualt Shunt Resistor" Shunt-Enum."Open" ("Shunt Resistor") Shunt-Enum."Open" ("Shunt Resistor")] -> w161
                    tunnel: [Input_Configuration-Enum."Differential" ("Input Configuation") Input_Configuration-Enum."Differential" ("Input Configuation") Input_Configuration-Enum."Differential" ("Input Configuation") Input_Configuration-Enum."Differential" ("Input Configuation") Input_Configuration-Enum."SE+ (-gnd)" ("Input Configuation")] -> w160
                    frame 0, Default {
                      # "Vsg - gate"
                    }
                    frame 1 {
                      # "Vbg - gate"
                    }
                    frame 2 {
                      # "I - current"
                    }
                    frame 3 {
                      # "dV - V (Diff)"
                    }
                    frame 4 {
                      # "V - V (SE)"
                    }
                  }
                }
              }
            }
            n76 = property on="Values have changed" class="Bool (strict)"("Val(Sgnl)"=TRUE ("Values have changed")) -> ()  [unwired: 2 in, 2 out]
            n77 = local read "Lockin"() -> (w139:T7)
            n78 = Bundle By Name(cluster=w139, "Electrode Config"=w137) -> (w138:T7)
            n79 = local read "KH"() -> (w136:T5)
            n80 = Bundle By Name(cluster=w136, "KH Shunt Resistor"=w134, "KH Configuration"=w135) -> (w133:T5)
            n81 = local write "Lockin"(w138) -> ()
            n82 = local write "KH"(w133) -> ()
            n83 = call <vilib>:"Add State(s) to Queue__jki_lib_state_machine.vi"("State(s) in (\"\")"=w145) -> ("States Out"=w144:string)  [unwired: 14 in]
          }
          event "KH.KH Shunt Resistor", "KH.KH Gain", "non KH.Electrodes 2", "non KH.Labels 2", "Sample (SAXXXX)", "Username", "Description", "Lockin.Electrode": Value Change {
            n84 = event-data() -> ()  [unwired: 1 in, 6 out]
            n85 = property on="Values have changed" class="Bool (strict)"("Val(Sgnl)"=TRUE ("Values have changed")) -> ()  [unwired: 2 in, 2 out]
          }
          event "Lockin.AI", "non KH.AO": Mouse Move; "Lockin.AI", "non KH.AO": Mouse Wheel {
            n86 = event-data() -> ()  [unwired: 1 in, 5 out]
            n87 = call <vilib>:"Add State(s) to Queue__jki_lib_state_machine.vi"("State(s) in Front (\"\")"="UI: Link Scroll Bars" ("State(s) in Front (\"\")"), "State(s) in (\"\")"=w185) -> ("States Out"=w184:string)  [unwired: 13 in]
          }
          event "#AI": Value Change {
            n88 = event-data() -> ("NewVal"=w194:u32)  [unwired: 1 in, 5 out]
            n89 = for {
              N: w194 -> [_]
              tunnel: [w203] -> w189 mode=indexing
              tunnel: [w202] -> w188 mode=indexing
              i -> [w202]
              n90 = Increment(x=w202) -> (x+1=w203:i32)
            }
            n91 = local read "Lockin"() -> (w197:T7)
            n92 = Bundle By Name(cluster=w197, "AI"=w189) -> (w196:T7)
            n93 = Initialize Array(1.0 ("element"), w194) -> (w192:dbl[])
            n94 = local read "KH"() -> (w191:T5)
            n95 = local write "Lockin"(w196) -> ()
            n96 = Bundle By Name(cluster=w191, "KH #"=w188) -> (w195:T5)
            n97 = local write "Gain"(w192) -> ()
            n98 = local write "KH"(w195) -> ()
            n99 = call <vilib>:"Add State(s) to Queue__jki_lib_state_machine.vi"("State(s) in Front (\"\")"="KH: set KH 0\nKH: set KH 1" ("State(s) in Front (\"\")"), "State(s) in (\"\")"=w200) -> ("States Out"=w199:string)  [unwired: 13 in]
          }
          event "KH Addresses": Value Change {
            n100 = event-data() -> ()  [unwired: 1 in, 6 out]
            n101 = local read "KH"() -> (w204:T5)
            n102 = Unbundle By Name(w204) -> ("KH #"=w206:u16[])
            n103 = Array Subset(array=w206) -> (w205:u16[])  [unwired: 2 in]
            n104 = Bundle By Name(cluster=w204, "KH #"=w205) -> (w207:T5)
            n105 = local write "KH"(w207) -> ()
            n106 = call <vilib>:"Add State(s) to Queue__jki_lib_state_machine.vi"("State(s) in Front (\"\")"="KH: set KH 0\nKH: set KH 1", "State(s) in (\"\")"=w212) -> ("States Out"=w211:string)  [unwired: 13 in]
          }
          event Panel Close? {
            # "Discard the event because we'll close the front panel ourselves in Macro: Exit"
            # "Close Panel button (pressed) Event\n(this executes Macro: Exit to terminate the VI)"
            n107 = event-data() -> ()  [unwired: 1 in, 1 out]
            n108 = event-data("Discard?"=TRUE) -> ()  [unwired: 1 in, 1 out]
            n109 = call <vilib>:"Add State(s) to Queue__jki_lib_state_machine.vi"("State(s) in Front (\"\")"="Macro: Exit", "State(s) in (\"\")"=w218) -> ("States Out"=w217:string)  [unwired: 13 in]
          }
        }
      }
      frame "---------- Core ----------" {
        # "Do not put any code in this frame.\n(it is a separator no-op)"
        n110 = call <vilib>:"Add State(s) to Queue__jki_lib_state_machine.vi"("State(s) in (\"\")"=w222) -> ("States Out"=w221:string)  [unwired: 14 in]
      }
      frame Default {
        w232 = 42 items=["No error", "Argument error", "Memory is full", "Out of zone", "End of file", "File already open", "Generic file I/O error", "File not found", "File permission error", "Disk is full", "Duplicate path", "Too many files open", "System feature not enabled", "Resource file not found", "Cannot add resource", "Resource not found", "Image not found", "Image memory error", "Pen does not exist", "Config type invalid", "Config token not found", "Config parse error", "Config memory error", "Bad external code format", "Bad external code offset", "External code not present", "Null window", "Destroy window error", "Null menu", "Print aborted", "Bad print record", "Print driver error", "Windows error during printing", "Memory error during printing", "Print dialog error", "Generic print error", "Invalid device refnum", "Device not found", "Device parameter error", "Device unit error", "Cannot open device", "Device call aborted", "Generic error", "Cancelled by user", "Object ID too low", "Object ID too high", "Object not in heap", "Unknown heap", "Unknown object (invalid DefProc)", "Unknown object (DefProc not in table)", "Message out of range", "Invalid (null) method", "Unknown message", "Manager call not supported", "Bad address", "Network operation in progress", "Network operation timed out", "Connection is busy", "Network attribute not supported", "Network error", "Address in use", "System out of memory", "Connection aborted", "Connection refused", "Not connected", "Already connected", "Connection closed", "Initialization error (interapplication manager)", "Bad occurrence", "Wait on unbound occurrence handler", "Occurrence queue overflow", "Datalog type conflict", "Unused", "Unrecognized type (interapplication manager)", "Memory corrupt", "Failed to make temporary DLL", "Old CIN version", "Drag socket not found", "Failed to load drop-object", "Failed to register OLE object", "Failed to release OLE object", "Format specifier type mismatch", "Unknown format specifier", "Too few format specifiers", "Too many format specifiers", "Scan failed", "Newer CIN version", "Error converting to variant", "Runtime menu error", "Password tampered", "Variant attribute not found", "Incompatible variant data type", "Event data is not available", "Event Store is not present", "Occurrence is not found", "Event Queue is not created", "Event info is not available", "Refnum passed is NULL", "Error retrieving Class GUID", "Error retrieving CoClass GUID", "Error retrieving TypeLib GUID.", "Bad built application magic bytes.", "Specific driver is different from the specific driver associated with the Logical Name.", "There is no session opened to the class driver.", "Max Error", "MAX - Error with config objects", "MAX - Error loading configuration", "MAX - Group not supported"]
        # "Current State"
        # "Do not delete, rename, or modify this frame.\n(this is used to capture unhandled states and typos)"
        # "Handle mistyped state name (developer tool)"
        n111 = Format Into String(format string="Software Exception: Unhandled State \"%s\"." ("message"), error in=w228, w223) -> (resulting string=w231:string, error out=w230:errorcluster)  [unwired: 1 in]
        n112 = call <vilib>:"Error Cluster From Error Code.vi"("show call chain? (False)"=TRUE, "error in (no error)"=w230, "error message (\"\")"=w231, "error code (0)"=w232) -> ("error out"=w229:errorcluster)  [unwired: 5 in]
        n113 = call <vilib>:"Add State(s) to Queue__jki_lib_state_machine.vi"("State(s) in (\"\")"=w227) -> ("States Out"=w226:string)  [unwired: 14 in]
      }
      frame "Initialize Core Data" {
        # "Do not delete, rename, or modify this frame.\n(this is used to determine panel behavior on exit)"
        # "originally closed?"
        # "exe?"
        # "If panel starts closed or is an EXE, then close it when we exit"
        n114 = property class="App"() -> ("App.Kind"=w240:T15)  [unwired: 2 in, 2 out]
        n115 = property class="VI"() -> ("Front Panel.Open"=w241:bool)  [unwired: 2 in, 2 out]
        n116 = control-ref of="Current VI Reference"() -> (w234:refnum<vi>)
        n117 = Not(x=w241) -> (.not. x?=w238:bool)
        n118 = Equal?(x=w240, y=T15."Run Time System" ("Application:Kind")) -> (x = y?=w237:bool)
        n119 = Or(x=w238, y=w237) -> (x .or. y?=w235:bool)
        n120 = Bundle By Name(cluster=w236, "Core.Current VI Reference"=w234, "Core.Close Panel on Exit?"=w235) -> (w243:T30)
        n121 = call <vilib>:"Add State(s) to Queue__jki_lib_state_machine.vi"("State(s) in (\"\")"=w245) -> ("States Out"=w244:string)  [unwired: 14 in]
      }
      frame "Error Handler" {
        # "Unhandled Error -- Display it"
        # "Handle any errors here.\nYou can also output any states to clean-up after errors occur"
        # "Clear error"
        n122 = call <vilib>:"General Error Handler.vi"("error in (no error)"=w247) -> ()  [unwired: 10 in, 5 out]
        n123 = call <vilib>:"Add State(s) to Queue__jki_lib_state_machine.vi"("State(s) in Front (\"\")"="/* Post Error States", "State(s) in (\"\")"=w251) -> ("States Out"=w250:string)  [unwired: 13 in]
      }
      frame "Exit" {
        # "Do not put any code in this frame.\n(No errors that occur here will be handled.)"
        n124 = call <vilib>:"Add State(s) to Queue__jki_lib_state_machine.vi"("State(s) in (\"\")"=w256) -> ("States Out"=w255:string)  [unwired: 14 in]
      }
      frame "---------- Data ----------" {
        # "Do not put any code in this frame.\n(It is a separator no-op. You can make a copy of this frame to create a new Data frame)"
        n125 = call <vilib>:"Add State(s) to Queue__jki_lib_state_machine.vi"("State(s) in (\"\")"=w260) -> ("States Out"=w259:string)  [unwired: 14 in]
      }
      frame "Data: Initialize" {
        w262 = path[] []  # VI paths
        w263 = refnum<class "Logger.PGSQL.lvclass"> refnum  # Logger
        w264 = T28 {"Sample"="", "Device"="", "Username"="", "Description"="", "Default Path"=path "", "AWS Path"=path "", "Instrument"=enum."----- AFM/EBL -----", "Lockin?"=FALSE, "Lockin Address"="", "Krohn Hite?"=FALSE, "KH Addresses"=[], "KH All Buttons"=enum."No Selection", "Strain Cell?"=FALSE, "Strain Cell Address"="", "C Bridge?"=FALSE, "Capacitance Bridge Address"="", "Lockin"={"AI"=[], "Electrode"=[], "Label"=[], "Electrode Config"=[]}, "KH"={"KH #"=[], "KH Configuration"=[], "KH Gain"=[], "KH Shunt Resistor"=[], "Filter"=FALSE, "DC Coupled"=FALSE}, "non KH"={"Scroll Bar"=[], "Electrodes 2"=[], "Labels 2"=[], "unused"=[]}, "#AI"=8}  # UI
        w270 = refnum<class "Configuration.lvclass"> refnum  # Config
        w273 = T31 {"Authentication Info"={"Client ID"="1150712142949183", "Client Secret"="530770942aed47201cd52aeb331bdd57", "Redirect URI"="https://www.google.com/", "Token Endpoint"="https://app.asana.com/-/oauth_token", "Scope"=""}, "Authentication Header"=[], "Refresh Token"="", "Time Stamp"=timestamp(0 s since 1904-01-01)}  # Asana
        w274 = cluster{"Channel Setting":T27}[] []  # Channel Settings
        w268 = T32 {"Current VI Reference"=refnum, "Close Panel on Exit?"=FALSE}  # Core
        # "Initialize the shift-register data, here.\n(data names are defined by what you wire into the bundle function)"
        n126 = local read "Refresh Token Out"() -> (w272:string)
        n127 = Unbundle By Name("C.E.") -> ("Experiment"=w275:T25, "Wiring Configuration"=w276:T26)
        n128 = Bundle By Name(cluster=w273, "Refresh Token"=w272) -> (w271:T31)
        n129 = Bundle("Core"=w268, "C.E."="C.E.", "Experiment"=w275, "Wiring Configuration"=w276, "Channel Settings"=w274, "KH All Buttons"="KH All Buttons", "Lockin"="Lockin", "KH"="KH", "non KH"="non KH", "UI"=w264, "Asana"=w271, "Logger"=w263, "Config"=w270, "VI paths"=w262) -> (w278:T30)  [unwired: 1 in]
        n130 = call <vilib>:"Add State(s) to Queue__jki_lib_state_machine.vi"("State(s) in (\"\")"=w280) -> ("States Out"=w279:string)  [unwired: 14 in]
      }
      frame "Data: Load Configuration" {
        w286 = T33 3 items=["User Home"=0, "User Desktop"=1, "User Documents"=2, "User Application Data"=3, "User Preferences"=4, "User Temporary"=5, "Public Documents"=6, "Public Application Data"=7, "Public Preferences"=8, "Public Cache"=13, "System Core Libraries"=9, "System Installed Libraries"=10, "Application Files"=11, "Boot Volume Root"=12] ("system directory type")
        n131 = disable-structure shown="Disabled" {
          frame Disabled {
            w304 = T33 7 items=["User Home"=0, "User Desktop"=1, "User Documents"=2, "User Application Data"=3, "User Preferences"=4, "User Temporary"=5, "Public Documents"=6, "Public Application Data"=7, "Public Preferences"=8, "Public Cache"=13, "System Core Libraries"=9, "System Installed Libraries"=10, "Application Files"=11, "Boot Volume Root"=12] ("system directory type")
            n132 = call <vilib>:"Get System Directory.vi"("system directory type"=w304) -> ("system directory"=w301:path)  [unwired: 10 in]
            n133 = Build Path(base path=w301, name or relative path="Levylab") -> (appended path=w303:path)
            n134 = Build Path(base path=w303, name or relative path="Control Experiment") -> ()  [unwired: 1 out]
          }
          frame Enabled {
          }
        }
        n135 = Unbundle By Name(w296) -> ("Config"=w298:refnum<class "Configuration.lvclass">, "UI"=w290:T28)
        n136 = call <vilib>:"Get System Directory.vi"("system directory type"=w286) -> ("system directory"=w285:path)  [unwired: 10 in]
        n137 = Build Path(base path=w285, name or relative path="LevyLab") -> (appended path=w283:path)
        n138 = Build Path(base path=w283, name or relative path="Control Experiment") -> (appended path=w281:path)
        n139 = call <userlib>:"Write Path.vi"("error in (no error)"=w297, "Path"=w281, "Configuration in"=w298) -> ("error out"=w293:errorcluster, "Configuration out"=w294:refnum<class "Configuration.lvclass">)  [unwired: 7 in]
        n140 = call <userlib>:"Read Configuration.vi"("INI Fomatted Cluster Type"=w290, "error in (no error)"=w293, "Configuration in"=w294) -> ("error out"=w292:errorcluster, "Configuration"=w288:variant, "Configuration out"=w289:refnum<class "Configuration.lvclass">)  [unwired: 6 in]
        n141 = Variant To Data(error in=w292, type=w290, Variant=w288) -> (data=w287:T28, error out=w291:errorcluster)
        n142 = Bundle By Name(cluster=w296, "Config"=w289, "UI"=w287) -> (w295:T30)
        n143 = call <vilib>:"Add State(s) to Queue__jki_lib_state_machine.vi"("State(s) in (\"\")"=w300) -> ("States Out"=w299:string)  [unwired: 14 in]
      }
      frame "Data: Save Controls" {
        n144 = local read "Sample (SAXXXX)"() -> (w336:string)
        n145 = local read "Default Path"() -> (w332:path)
        n146 = local read "Username"() -> (w334:string)
        n147 = local read "Strain Cell?"() -> (w326:bool)
        n148 = local read "C Bridge?"() -> (w324:bool)
        n149 = local read "Lockin"() -> (w322:T7)
        n150 = local read "Lockin Address"() -> (w330:string)
        n151 = local read "KH Addresses"() -> (w328:refnum<visa-resource-name>[])
        n152 = local read "KH"() -> (w315:T5)
        n153 = local read "Description"() -> (w333:string)
        n154 = local read "Strain Cell Address"() -> (w325:refnum<visa-resource-name>)
        n155 = local read "Capacitance Bridge Address"() -> (w323:refnum<visa-resource-name>)
        n156 = local read "Instrument"() -> (w331:T9)
        n157 = Unbundle By Name(w315) -> ("KH #"=w314:u16[], "KH Configuration"=w311:T2[], "KH Gain"=w312:T3[], "KH Shunt Resistor"=w313:T4[])
        n158 = local read "Device (YYYYMMDD)"() -> (w335:string)
        n159 = local read "Krohn Hite?"() -> (w329:bool)
        n160 = local read "KH All Buttons"() -> (w327:T8)
        n161 = local read "AWS Credentials"() -> (w307:path)
        n162 = local read "non KH"() -> (w316:T10)
        n163 = local read "#AI"() -> (w306:u32)
        n164 = Bundle By Name(cluster=w317, "UI.Sample"=w336, "UI.Device"=w335, "UI.Username"=w334, "UI.Description"=w333, "UI.Default Path"=w332, "UI.AWS Path"=w307, "UI.Instrument"=w331, "UI.Lockin Address"=w330, "UI.Krohn Hite?"=w329, "UI.KH Addresses"=w328, "UI.KH All Buttons"=w327, "UI.Strain Cell?"=w326, "UI.Strain Cell Address"=w325, "UI.C Bridge?"=w324, "UI.Capacitance Bridge Address"=w323, "UI.Lockin"=w322, "UI.non KH"=w316, "UI.KH.KH #"=w314, "UI.KH.KH Configuration"=w311, "UI.KH.KH Gain"=w312, "UI.KH.KH Shunt Resistor"=w313, "UI.KH.Filter"="Bandwidth Filter", "UI.KH.DC Coupled"="DC Coupled", "UI.#AI"=w306) -> (w308:T30)
        n165 = Unbundle By Name(w308) -> ("Config"=w321:refnum<class "Configuration.lvclass">, "UI"=w320:T28)
        n166 = call <userlib>:"Write Configuration.vi"("error in (no error)"=w319, "Variant"=w320, "Configuration in"=w321) -> ("error out"=w318:errorcluster)  [unwired: 7 in, 1 out]
        n167 = call <vilib>:"Add State(s) to Queue__jki_lib_state_machine.vi"("State(s) in (\"\")"=w338) -> ("States Out"=w337:string)  [unwired: 14 in]
      }
      frame "Data: Cleanup" {
        # "Cleanup any data and references, here.\n(this is called automatically, by the Macro: Exit)"
        n168 = Unbundle By Name(w341) -> ("Core.Current VI Reference"=w340:refnum<vi>, "Logger"=w343:refnum<class "Logger.PGSQL.lvclass">)
        n169 = call <vilib>:"Stop.vi"("error in (no error)"=w342, "SMO"=w343) -> ("error out"=w339:errorcluster)  [unwired: 8 in, 1 out]
        n170 = Close Reference(reference=w340, error in (no error)=w339) -> (error out=w344:errorcluster)
        n171 = call <vilib>:"Add State(s) to Queue__jki_lib_state_machine.vi"("State(s) in (\"\")"=w346) -> ("States Out"=w345:string)  [unwired: 14 in]
      }
      frame "---------- UI ----------" {
        # "Do not put any code in this frame.\n(It is a separator no-op. You can make a copy of this frame to create a new UI frame)"
        n172 = call <vilib>:"Add State(s) to Queue__jki_lib_state_machine.vi"("State(s) in (\"\")"=w350) -> ("States Out"=w349:string)  [unwired: 14 in]
      }
      frame "UI: Initialize" {
        w352 = TRUE ("Visible")
        (unwired) string[] ["", "I+", "I-", "V1+", "V1-", "V2+", "V2-", "V3+", "V3-", "V4+", "V4-", "dV1", "dV2", "dV3", "Vsg", "Vbg"] ("Strings [] 2")
        # "Pickering? = False always"
        # "unused"
        # "Initialize the User Interface, here.\n(this is called automatically, by the Macro: Init)"
        n173 = local read "Labels Strings"() -> (w363:string[])
        n174 = call <userlib>:"Fit VI window to Largest Dec__ogtk.vi"("error in (no error)"=w368) -> ("error out"=w365:errorcluster)  [unwired: 5 in, 1 out]
        n175 = Unbundle By Name(w358) -> ("UI.Krohn Hite?"=w355:bool, "UI.Strain Cell?"=w354:bool, "UI.C Bridge?"=w353:bool)
        n176 = property on="OK" class="Bool (strict)"("Value"=FALSE ("Blinking")) -> ()  [unwired: 2 in, 2 out]
        n177 = property on="Ring" class="Ring (strict)"(error in=w365, "Strings []"=w363) -> (error out=w364:errorcluster)  [unwired: 1 in, 1 out]
        n178 = local write "KH All Buttons"(T8."No Selection" ("KH All Buttons")) -> ()
        n179 = property on="Values have changed" class="Bool (strict)"("Val(Sgnl)"=TRUE ("Blinking")) -> ()  [unwired: 2 in, 2 out]
        n180 = property on="Ring" class="Ring (strict)"(error in=w364, "Strings []"=w363) -> (error out=w366:errorcluster)  [unwired: 1 in, 1 out]
        n181 = property on="Tab Control" class="TabCtl (strict)"("Value"=T1."Input" ("Tab Control")) -> ()  [unwired: 2 in, 2 out]
        n182 = property on="Krohn Hite?" class="Bool (strict)"("Val(Sgnl)"=w355, "Visible"=w352) -> ()  [unwired: 2 in, 2 out]
        n183 = disable-structure shown="Enabled" {
          disable-tunnel: w366 -> [w373 w374]
          disable-tunnel: [w372 w374] -> w359
          disable-tunnel: FALSE ("Blinking") -> [w371 _]
          frame Disabled {
            n184 = property on="Pickering?" class="Bool (strict)"(error in=w373, "Val(Sgnl)"=w371) -> (error out=w372:errorcluster)  [unwired: 1 in, 1 out]
          }
          frame Enabled {
          }
        }
        n185 = property on="#AI" class="DigNum (strict)"("Val(Sgnl)"="#AI") -> ()  [unwired: 2 in, 2 out]
        n186 = property on="Strain Cell?" class="Bool (strict)"("Val(Sgnl)"=w354, "Visible"=w352) -> ()  [unwired: 2 in, 2 out]
        n187 = local read "KH Addresses"() -> (w356:refnum<visa-resource-name>[])
        n188 = property on="C Bridge?" class="Bool (strict)"("Val(Sgnl)"=w353, "Visible"=w352) -> ()  [unwired: 2 in, 2 out]
        n189 = property on="KH Addresses" class="Arr (strict)"("Val(Sgnl)"=w356) -> ()  [unwired: 2 in, 2 out]
        n190 = call <vilib>:"Add State(s) to Queue__jki_lib_state_machine.vi"("State(s) in (\"\")"=w370) -> ("States Out"=w369:string)  [unwired: 14 in]
      }
      frame "UI: Update Controls" {
        # "Do not put any code in this frame.\n(It is a separator no-op. You can make a copy of this frame to create a new Data frame)"
        n191 = Unbundle By Name(w377) -> ("UI.Sample"=w393:string, "UI.Device"=w394:string, "UI.Username"=w395:string, "UI.Description"=w396:string, "UI.Default Path"=w401:path, "UI.AWS Path"=w376:path, "UI.Instrument"=w397:T9, "UI.Lockin Address"=w391:string, "UI.Krohn Hite?"=w400:bool, "UI.KH Addresses"=w392:refnum<visa-resource-name>[], "UI.KH All Buttons"=w388:T8, "UI.Strain Cell?"=w399:bool, "UI.Strain Cell Address"=w389:refnum<visa-resource-name>, "UI.C Bridge?"=w398:bool, "UI.Capacitance Bridge Address"=w390:refnum<visa-resource-name>, "UI.Lockin"=w387:T7, "UI.non KH"=w386:T34, "UI.KH.Filter"=w384:bool, "UI.KH.DC Coupled"=w385:bool, "UI.KH.KH #"=w381:T24, "UI.KH.KH Configuration"=w380:T2[], "UI.KH.KH Gain"=w379:T3[], "UI.KH.KH Shunt Resistor"=w378:T4[], "UI.#AI"=w375:u32)
        n192 = local write "Sample (SAXXXX)"(w393) -> ()
        n193 = local write "Krohn Hite?"(w400) -> ()
        n194 = local write "Bandwidth Filter"(w384) -> ()
        n195 = local write "Strain Cell?"(w399) -> ()
        n196 = local write "C Bridge?"(w398) -> ()
        n197 = local write "Username"(w395) -> ()
        n198 = local write "Lockin"(w387) -> ()
        n199 = local write "Instrument"(w397) -> ()
        n200 = local write "Default Path"(w401) -> ()
        n201 = local write "Strain Cell Address"(w389) -> ()
        n202 = local write "KH Addresses"(w392) -> ()
        n203 = local write "Capacitance Bridge Address"(w390) -> ()
        n204 = local write "DC Coupled"(w385) -> ()
        n205 = local write "non KH"(w386) -> ()
        n206 = local write "#AI"(w375) -> ()
        n207 = local write "Device (YYYYMMDD)"(w394) -> ()
        n208 = local write "AWS Credentials"(w376) -> ()
        n209 = local write "Description"(w396) -> ()
        n210 = local write "Lockin Address"(w391) -> ()
        n211 = local write "KH All Buttons"(w388) -> ()
        n212 = local read "KH"() -> (w383:T5)
        n213 = Bundle By Name(cluster=w383, "KH #"=w381, "KH Configuration"=w380, "KH Gain"=w379, "KH Shunt Resistor"=w378) -> (w382:T5)
        n214 = local write "KH"(w382) -> ()
        n215 = call <vilib>:"Add State(s) to Queue__jki_lib_state_machine.vi"("State(s) in (\"\")"=w404) -> ("States Out"=w403:string)  [unwired: 14 in]
      }
      frame "UI: Cursor Set" {
        # "Argument"
        # "Set and Unset Cursor Busy.\n(Usage: \"UI: Cursor Set >> Busy|Idle\")"
        n216 = case shown="\"Busy\"" w405 {
          tunnel: w407 -> [w412 w414]
          tunnel: [w411 w413] -> w406
          frame "Idle", Default {
            n217 = call <vilib>:"Unset Busy.vi"("error in (no error)"=w412) -> ("error out"=w411:errorcluster)  [unwired: 10 in]
          }
          frame "Busy" {
            n218 = call <vilib>:"Set Busy.vi"("error in (no error)"=w414) -> ("error out"=w413:errorcluster)  [unwired: 9 in, 1 out]
          }
        }
        n219 = call <vilib>:"Add State(s) to Queue__jki_lib_state_machine.vi"("State(s) in (\"\")"=w410) -> ("States Out"=w409:string)  [unwired: 14 in]
      }
      frame "UI: Front Panel State" {
        # "Argument"
        # "Set Front Panel Open or Closed\n(Usage: \"UI: Front Panel State >> Open|Close\")"
        n220 = Unbundle By Name(w417) -> ("Core.Current VI Reference"=w416:refnum<vi>)
        n221 = case shown="\"Open\", Default" w415 {
          tunnel: w419 -> [w425 w438]
          tunnel: [w427 w439] -> w418
          tunnel: w416 -> [w426 w436]
          frame "Open", Default {
            n222 = property class="VI"(reference=w426, error in=w425) -> (reference out=w423:refnum<vi>, error out=w424:errorcluster, "Front Panel.Open"=w422:bool)
            n223 = case shown="True" w422 {
              tunnel: [w430 w433] -> w427
              tunnel: w424 -> [w429 w433]
              tunnel: w423 -> [w428 _]
              frame False {
                n224 = invoke class="VI" method="FP.Open"(reference=w428, error in=w429, "Activate"=TRUE, "State"=T16."Standard") -> (error out=w430:errorcluster)  [unwired: 1 in, 4 out]
              }
              frame True {
              }
            }
          }
          frame "Close" {
            n225 = property class="VI"(reference=w436, error in=w438) -> (reference out=w435:refnum<vi>, error out=w437:errorcluster, "Front Panel.Open"=w434:bool)
            n226 = case shown="True" w434 {
              tunnel: [w440 w443] -> w439
              tunnel: w437 -> [w440 w442]
              tunnel: w435 -> [_ w441]
              frame False {
              }
              frame True {
                n227 = invoke class="VI" method="FP.Close"(reference=w441, error in=w442) -> (error out=w443:errorcluster)  [unwired: 1 in, 2 out]
              }
            }
          }
        }
        n228 = call <vilib>:"Add State(s) to Queue__jki_lib_state_machine.vi"("State(s) in (\"\")"=w421) -> ("States Out"=w420:string)  [unwired: 14 in]
      }
      frame "UI: Buttons" {
        # "Do not put any code in this frame.\n(It is a separator no-op. You can make a copy of this frame to create a new UI frame)"
        n229 = call <vilib>:"Add State(s) to Queue__jki_lib_state_machine.vi"("State(s) in (\"\")"=w447) -> ("States Out"=w446:string)  [unwired: 14 in]
      }
      frame "UI: Link Scroll Bars" {
        # "Do not put any code in this frame.\n(It is a separator no-op. You can make a copy of this frame to create a new UI frame)"
        n230 = control-ref of="AI"() -> (w458:refnum<vi>)
        n231 = control-ref of="Electrode"() -> (w457:refnum<vi>)
        n232 = control-ref of="Label"() -> (w456:refnum<vi>)
        n233 = control-ref of="Electrode Config"() -> (w455:refnum<vi>)
        n234 = control-ref of="KH #"() -> (w454:refnum<vi>)
        n235 = control-ref of="KH Configuration"() -> (w453:refnum<vi>)
        n236 = control-ref of="KH Gain"() -> (w452:refnum<vi>)
        n237 = control-ref of="KH Shunt Resistor"() -> (w451:refnum<vi>)
        n238 = control-ref of="Gain"() -> (w449:refnum<vi>)
        n239 = property class="Arr (strict)"(reference=w458) -> ("Index Values"=w448:u32[])  [unwired: 1 in, 2 out]
        n240 = property class="Arr (strict)"(reference=w457, "Index Values"=w448) -> ()  [unwired: 1 in, 2 out]
        n241 = property class="Arr (strict)"(reference=w456, "Index Values"=w448) -> ()  [unwired: 1 in, 2 out]
        n242 = property class="Arr (strict)"(reference=w455, "Index Values"=w448) -> ()  [unwired: 1 in, 2 out]
        n243 = property class="Arr (strict)"(reference=w454, "Index Values"=w448) -> ()  [unwired: 1 in, 2 out]
        n244 = property class="Arr (strict)"(reference=w453, "Index Values"=w448) -> ()  [unwired: 1 in, 2 out]
        n245 = property class="Arr (strict)"(reference=w452, "Index Values"=w448) -> ()  [unwired: 1 in, 2 out]
        n246 = property class="Arr (strict)"(reference=w451, "Index Values"=w448) -> ()  [unwired: 1 in, 2 out]
        n247 = property class="Arr (strict)"(reference=w449, "Index Values"=w448) -> ()  [unwired: 1 in, 2 out]
        n248 = property on="AO" class="Arr (strict)"() -> ("Index Values"=w450:u32[])  [unwired: 2 in, 2 out]
        n249 = property on="Labels 2" class="Arr (strict)"("Index Values"=w450) -> ()  [unwired: 2 in, 2 out]
        n250 = property on="unused" class="Arr (strict)"("Index Values"=w450) -> ()  [unwired: 2 in, 2 out]
        n251 = property on="Electrodes 2" class="Arr (strict)"("Index Values"=w450) -> ()  [unwired: 2 in, 2 out]
        n252 = call <vilib>:"Add State(s) to Queue__jki_lib_state_machine.vi"("State(s) in (\"\")"=w462) -> ("States Out"=w461:string)  [unwired: 14 in]
      }
      frame "UI: SR Disable" {
        # "Do not put any code in this frame.\n(It is a separator no-op. You can make a copy of this frame to create a new UI frame)"
        n253 = local read "KH Addresses"() -> (w472:refnum<visa-resource-name>[])
        n254 = control-ref of="Shunt Resistor"() -> (w468:refnum<vi>)
        n255 = Index Array(array=w472) -> (element=w471:refnum<visa-resource-name>)  [unwired: 1 in]
        n256 = call <userlib>:"Shunt - Check 500 or 10M.vi"("error in (no error)"=w470, "VISA Refnum in"=w471) -> ("error out"=w469:errorcluster, "SR"=w465:enum16{"500", "10M"})  [unwired: 7 in, 1 out]
        n257 = call <vilib>:"Clear Errors.vi"("error in (no error)"=w469) -> ("error out"=w467:errorcluster)  [unwired: 5 in, 1 out]
        n258 = call <userlib>:"Shunt - 500 or 10M Control Disable.vi"("error in"=w467, "SR"=w465, "reference"=w468) -> ("error out"=w464:errorcluster)  [unwired: 8 in]
        n259 = control-ref of="Defualt Shunt Resistor"() -> (w466:refnum<vi>)
        n260 = call <userlib>:"Shunt - 500 or 10M Control Disable.vi"("error in"=w464, "SR"=w465, "reference"=w466) -> ("error out"=w463:errorcluster)  [unwired: 8 in]
        n261 = call <vilib>:"Add State(s) to Queue__jki_lib_state_machine.vi"("State(s) in (\"\")"=w475) -> ("States Out"=w474:string)  [unwired: 14 in]
      }
      frame "---------- Macro ----------" {
        # "Do not put any code in this frame.\n(It is a separator no-op. You can make a copy of this frame to create a new Macro frame)"
        n262 = call <vilib>:"Add State(s) to Queue__jki_lib_state_machine.vi"("State(s) in (\"\")"=w479) -> ("States Out"=w478:string)  [unwired: 14 in]
      }
      frame "Macro: Initialize" {
        # "Initialization Macro\n(This is called once, when the VI starts)"
        n263 = call <vilib>:"Add State(s) to Queue__jki_lib_state_machine.vi"("State(s) in Front (\"\")"="Data: Initialize\nInitialize Core Data\nData: Load Configuration\nUI: Update Controls\nUI: Initialize\nUI: Front Panel State >> Open\nUI: SR Disable\nExperiment VI: Populate VI Ring\n//Asana: Initialize Authentication Info\n//Macro: Asana\nPGSQL: Start Logger", "State(s) in (\"\")"=w484) -> ("States Out"=w483:string)  [unwired: 13 in]
      }
      frame "Macro: Exit" {
        # "Exit Macro\n(This is called once, when the VI exits)"
        n264 = Unbundle By Name(w492) -> ("Core.Close Panel on Exit?"=w491:bool)
        n265 = property on="OK" class="Bool (strict)"("Value"=FALSE ("Blinking")) -> ()  [unwired: 2 in, 2 out]
        n266 = Select(t="UI: Front Panel State >> Close", s=w491, f="") -> (s? t:f=w488:string)
        n267 = call <vilib>:"Add State(s) to Queue__jki_lib_state_machine.vi"("State(s) in (\"\")"=w488, "State(s) at Back (\"\")"="Data: Save Controls\nData: Cleanup\nExit") -> ("States Out"=w486:string)  [unwired: 13 in]
        n268 = call <vilib>:"Add State(s) to Queue__jki_lib_state_machine.vi"("State(s) in Front (\"\")"=w486, "State(s) in (\"\")"=w495) -> ("States Out"=w494:string)  [unwired: 13 in]
      }
      frame "Macro: Output" {
        n269 = case shown="False" "I'm Finished Taking Data!" {
          tunnel: [w507 _] -> w499
          frame False {
            n270 = local read "Pickering?"() -> (w503:bool)
            n271 = case shown="False" w503 {
              tunnel: [w509 "Pickering: set Pickering" ("State(s) in Front (\"\")")] -> w504
              frame False {
                n272 = local read "KH Addresses"() -> (w512:refnum<visa-resource-name>[])
                n273 = Empty Array?(array=w512) -> (empty?=w511:bool)
                n274 = Select(t="", s=w511, f="UI: SR Disable\nKH: set KH 0\nKH: set KH 1\nKH: set KH 2" ("State(s) in Front (\"\")")) -> (s? t:f=w509:string)
              }
              frame True {
              }
            }
            n275 = call <vilib>:"Add State(s) to Queue__jki_lib_state_machine.vi"("State(s) in Front (\"\")"="Macro: Initialize Metadata" ("State(s) in Front (\"\")"), "State(s) in (\"\")"=w504, "State(s) at Back (\"\")"="Macro: Write Metadata" ("State(s) in Front (\"\")")) -> ("States Out"=w507:string)  [unwired: 12 in]
          }
          frame True {
          }
        }
        n276 = call <vilib>:"Add State(s) to Queue__jki_lib_state_machine.vi"("State(s) in Front (\"\")"=w499, "State(s) in (\"\")"=w502, "State(s) at Back (\"\")"="PGSQL: Write" ("State(s) in Front (\"\")")) -> ("States Out"=w501:string)  [unwired: 12 in]
      }
      frame "Macro: Initialize Metadata" {
        # "Do not put any code in this frame.\n(It is a separator no-op. You can make a copy of this frame to create a new Macro frame)"
        n277 = call <vilib>:"Add State(s) to Queue__jki_lib_state_machine.vi"("State(s) in Front (\"\")"="Metadata: Update Experiment Description\nMetadata: Update Wiring Configuration\nMetadata: Update KH\nMetadata: Build Path\nMetadata: Update Control Experiment Wire\nInstruments: Load Classes\nInstruments: Initialize KH\nInstruments: Initialize Lockin\nInstruments: Initialize Instruments" ("State(s) in Front (\"\")"), "State(s) in (\"\")"=w518) -> ("States Out"=w517:string)  [unwired: 13 in]
      }
      frame "Macro: Write Metadata" {
        # "Do not put any code in this frame.\n(It is a separator no-op. You can make a copy of this frame to create a new Macro frame)"
        n278 = call <vilib>:"Add State(s) to Queue__jki_lib_state_machine.vi"("State(s) in Front (\"\")"="Metadata: Update Comments\nMetadata: Write JSON\nMetadata: Update FGV\n//Macro: Asana" ("State(s) in Front (\"\")"), "State(s) in (\"\")"=w523) -> ("States Out"=w522:string)  [unwired: 13 in]
      }
      frame "Macro: Asana" {
        # "Do not put any code in this frame.\n(It is a separator no-op. You can make a copy of this frame to create a new Macro frame)"
        n279 = call <vilib>:"Add State(s) to Queue__jki_lib_state_machine.vi"("State(s) in Front (\"\")"="Asana: Authenticate\nAsana: Get Teams and Projects" ("State(s) in Front (\"\")"), "State(s) in (\"\")"=w528) -> ("States Out"=w527:string)  [unwired: 13 in]
      }
      frame "---------- Metadata ----------" {
        n280 = call <vilib>:"Add State(s) to Queue__jki_lib_state_machine.vi"("State(s) in (\"\")"=w532) -> ("States Out"=w531:string)  [unwired: 14 in]
      }
      frame "Metadata: Update Experiment Description" {
        n281 = Concatenate Strings("Sample (SAXXXX)", "." ("string"), "Device (YYYYMMDD)") -> (w536:string)
        n282 = Bundle By Name(cluster=w540, "Experiment.Device"=w536, "Experiment.User"="Username", "Experiment.Device Description"="Description", "Experiment.Instrument"="Instrument") -> (w541:T30)
        n283 = call <vilib>:"Add State(s) to Queue__jki_lib_state_machine.vi"("State(s) in (\"\")"=w544) -> ("States Out"=w543:string)  [unwired: 14 in]
      }
      frame "Metadata: Update Wiring Configuration" {
        n284 = local read "Lockin"() -> (w553:T7)
        n285 = local read "non KH"() -> (w547:T10)
        n286 = local read "Lockin"() -> (w551:T7)
        n287 = Unbundle By Name(w547) -> ("Electrodes 2"=w546:string[], "Labels 2"=w545:u16[])
        n288 = Unbundle By Name(w551) -> ("Electrode Config"=w550:T6[])
        n289 = Unbundle By Name(w553) -> ("AI"=w548:u32[], "Electrode"=w549:string[], "Label"=w552:u16[])
        n290 = for {
          tunnel: w545 -> [w562] mode=indexing
          tunnel: [w561] -> w554 mode=indexing
          n291 = property on="Ring" class="Ring (strict)"() -> ("Strings []"=w563:string[])  [unwired: 2 in, 2 out]
          n292 = Index Array(array=w563, index=w562) -> (element=w561:string)
        }
        n293 = for {
          tunnel: w552 -> [w565] mode=indexing
          tunnel: [w564] -> w555 mode=indexing
          n294 = property on="Ring" class="Ring (strict)"() -> ("Strings []"=w566:string[])  [unwired: 2 in, 2 out]
          n295 = Index Array(array=w566, index=w565) -> (element=w564:string)
        }
        n296 = Bundle By Name(cluster=w556, "Wiring Configuration.Lockin Ch"=w548, "Wiring Configuration.KH.Electrodes"=w549, "Wiring Configuration.KH.Labels"=w555, "Wiring Configuration.not KH.Electrodes"=w546, "Wiring Configuration.not KH.Labels"=w554, "Lockin.Electrode Config"=w550) -> (w557:T30)
        n297 = call <vilib>:"Add State(s) to Queue__jki_lib_state_machine.vi"("State(s) in (\"\")"=w560) -> ("States Out"=w559:string)  [unwired: 14 in]
      }
      frame "Metadata: Update KH" {
        n298 = local read "KH All Buttons"() -> (w580:T8)
        n299 = local read "KH"() -> (w582:T5)
        n300 = Unbundle By Name(w582) -> ("KH #"=w569:u16[], "KH Gain"=w579:T3[], "KH Configuration"=w568:T2[], "KH Shunt Resistor"=w576:T4[])
        n301 = call "Initialize KH Array.vi"("KH #"=w569, "Control in"=w579) -> ("Control out"=w581:variant)  [unwired: 9 in]
        n302 = Variant To Data(error in=w573, type=w579, Variant=w581) -> (data=w578:T3[], error out=w572:errorcluster)
        n303 = call "Initialize KH Array.vi"("KH #"=w569, "Control in"=w568) -> ("Control out"=w577:variant)  [unwired: 9 in]
        n304 = Variant To Data(error in=w572, type=w568, Variant=w577) -> (data=w567:T2[], error out=w571:errorcluster)
        n305 = call "Initialize KH Array.vi"("KH #"=w569, "Control in"=w576) -> ("Control out"=w574:variant)  [unwired: 9 in]
        n306 = Variant To Data(error in=w571, type=w576, Variant=w574) -> (data=w575:T4[], error out=w570:errorcluster)
        n307 = Bundle By Name(cluster=w583, "KH.KH #"=w569, "KH.KH Gain"=w578, "KH.KH Configuration"=w567, "KH.KH Shunt Resistor"=w575, "KH All Buttons"=w580) -> (w584:T30)
        n308 = call <vilib>:"Add State(s) to Queue__jki_lib_state_machine.vi"("State(s) in (\"\")"=w586) -> ("States Out"=w585:string)  [unwired: 14 in]
      }
      frame "Metadata: Build Path" {
        n309 = Unbundle By Name(w598) -> ("Experiment.Instrument"=w595:T9, "Experiment.Device"=w594:string)
        n310 = Format Into String(w595) -> (resulting string=w587:string)  [unwired: 3 in, 1 out]
        n311 = Build Path(base path="Default Path", name or relative path=w587) -> (appended path=w596:path)
        n312 = Build Path(base path=w596, name or relative path=w594) -> (appended path=w593:path)
        n313 = call <userlib>:"MGI Create Directory Chain.vi"("Error In"=w592, "File Presence (Auto Detect)"=MGI_Create_Directory_Chain_Behavior_Enum."Path Does Not Contain a File", "Path"=w593) -> ("Error Out"=w591:errorcluster, "Duplicate Path"=w589:path)  [unwired: 7 in]
        "Device Folder" <- w589
        n314 = Bundle By Name(cluster=w598, "Experiment.Device Path"=w589) -> (w597:T30)
        n315 = call <vilib>:"Add State(s) to Queue__jki_lib_state_machine.vi"("State(s) in (\"\")"=w600) -> ("States Out"=w599:string)  [unwired: 14 in]
      }
      frame "Metadata: Update Control Experiment Wire" {
        # "IS Control Experiment Class wire"
        # "Not on Control Experiment Class wire"
        n316 = call-poly <userlib>:"File Exists__ogtk.vi"("file path"="AWS Credentials") -> ("exists"=w603:bool)  [unwired: 6 in, 1 out]
        n317 = First Call?() -> (First Call?: T/F=w604:bool)
        n318 = Not(x=w603) -> (.not. x?=w601:bool)
        n319 = And(x=w601, y=w604) -> (x .and. y?=w602:bool)
        n320 = case shown="True" w602 {
          tunnel: "AWS Credentials" -> [w617 _]
          tunnel: [w617 _] -> w606
          tunnel: "https://docs.aws.amazon.com/cli/latest/userguide/cli-configure-files.html" ("URL") -> [_ w618]
          frame False {
          }
          frame True {
            n321 = call "Display Message to User"() -> ("OK"=w619:bool)  [unwired: 10 in, 1 out]
            n322 = case shown="True" w619 {
              tunnel: w618 -> [_ w620]
              frame False {
              }
              frame True {
                n323 = call-poly <vilib>:"Open URL in Default Browser.vi"("URL"=w620) -> ()  [unwired: 5 in, 2 out]
              }
            }
          }
        }
        n324 = Unbundle By Name(w612) -> ("C.E."=w610:refnum<class "Control Experiment SM.lvclass">, "Experiment"=w614:T25, "Wiring Configuration"=w613:T26)
        n325 = Bundle By Name(cluster=w610, "Experiment"=w614, "Wiring Configuration"=w613, "AWS Credentials"=w606) -> (w608:refnum<class "Control Experiment SM.lvclass">)
        n326 = Bundle By Name(cluster=w612, "C.E."=w608) -> (w611:T30)
        n327 = call <vilib>:"Add State(s) to Queue__jki_lib_state_machine.vi"("State(s) in (\"\")"=w616) -> ("States Out"=w615:string)  [unwired: 14 in]
      }
      frame "Metadata: Update Comments" {
        # "error 63 occurs when\nthe lockin isn't running\nI think we can clear here?"
        n328 = Unbundle By Name(w631) -> ("C.E."=w627:refnum<class "Control Experiment SM.lvclass">)
        n329 = call "Generate Comments.vi"("error in (no error)"=w622, "Control Experiment"=w627) -> ("error out"=w624:errorcluster, "Control Experiment out"=w626:refnum<class "Control Experiment SM.lvclass">)  [unwired: 6 in, 1 out]
        n330 = call <vilib>:"Clear Errors.vi"("error in (no error)"=w624, "specific error code to clear (0: all)"=63) -> ("error out"=w623:errorcluster)  [unwired: 4 in, 1 out]
        n331 = call "Read Comments.vi"("error in (no error)"=w623, "Control Experiment in"=w626) -> ("error out"=w621:errorcluster, "Comments"=→"Comments":string, "Control Experiment out"=w628:refnum<class "Control Experiment SM.lvclass">)  [unwired: 7 in]
        n332 = Bundle By Name(cluster=w631, "C.E."=w628) -> (w630:T30)
        n333 = call <vilib>:"Add State(s) to Queue__jki_lib_state_machine.vi"("State(s) in (\"\")"=w633) -> ("States Out"=w632:string)  [unwired: 14 in]
      }
      frame "Metadata: Update FGV" {
        n334 = Unbundle By Name(w638) -> ("C.E."=w635:refnum<class "Control Experiment SM.lvclass">)
        n335 = call "Control Experiment FGV.vi"("Function"=enum16{"read", "write"}."write", "error in (no error)"=w634, "Control Experiment.lvclass"=w635) -> ("error out"=w636:errorcluster)  [unwired: 7 in, 1 out]
        n336 = call <vilib>:"Add State(s) to Queue__jki_lib_state_machine.vi"("State(s) in (\"\")"=w640) -> ("States Out"=w639:string)  [unwired: 14 in]
      }
      frame "Metadata: Write JSON" {
        w651 = T35 {"Device"={"Device"="", "User"="", "Time"="", "Computer Name"=""}, "Wiring"={"Lockin Ch"=[], "KH Electrodes"=[], "KH Labels"=[], "Other Electrodes"=[], "Other Labels"=[]}}  # Control Experiment JSON
        n337 = Unbundle By Name(w643) -> ("C.E."=w652:refnum<class "Control Experiment SM.lvclass">, "Experiment.Device"=w667:string, "Experiment.User"=w666:string)
        n338 = Unbundle By Name(w643) -> ("Lockin.AI"=w665:u32[], "Wiring Configuration.KH.Electrodes"=w664:string[], "Wiring Configuration.KH.Labels"=w663:string[], "Wiring Configuration.KH.Electrodes"=w661:string[], "Wiring Configuration.KH.Labels"=w660:string[])
        n339 = call "Get Date Time ISO.vi"("error in (no error)"=w659) -> ("error out"=w656:errorcluster, "ISO 8601 date-time string"=w657:string)  [unwired: 8 in, 1 out]
        n340 = call "GetLocalComputerName.vi"("error in (no error)"=w656) -> ("error out"=w658:errorcluster, "Name"=w662:string)  [unwired: 8 in, 1 out]
        n341 = Bundle By Name(cluster=w651, "Device.Device"=w667, "Device.User"=w666, "Device.Time"=w657, "Device.Computer Name"=w662) -> (w650:T35)
        n342 = Bundle By Name(cluster=w650, "Wiring.Lockin Ch"=w665, "Wiring.KH Electrodes"=w664, "Wiring.KH Labels"=w663, "Wiring.Other Electrodes"=w661, "Wiring.Other Labels"=w660) -> (w649:T35)
        n343 = call <vilib>:"Flatten To JSON String.vi"("Enums As String (F)"=TRUE, "error in (no error)"=w658, "Variant"=w649) -> ("error out"=w654:errorcluster, "JSON String"=→"JSON String":string)  [unwired: 7 in]
        n344 = call "Write Experiment Folder.vi"("error in (no error)"=w654, "Experiment Folder"="device", "Control Experiment in"=w652) -> ("error out"=w653:errorcluster, "Control Experiment out"=w655:refnum<class "Control Experiment SM.lvclass">)  [unwired: 7 in]
        n345 = call "Save JSON File.vi"("error in (no error)"=w653, "Data"=w649, "Control Experiment in"=w655) -> ("error out"=w645:errorcluster, "JSON String"=w646:string, "Control Experiment out"=w647:refnum<class "Control Experiment SM.lvclass">)  [unwired: 6 in]
        n346 = call "Write Device Description JSON.vi"("error in (no error)"=w645, "Device Description JSON"=w646, "Control Experiment in"=w647) -> ("error out"=w644:errorcluster, "Control Experiment out"=w641:refnum<class "Control Experiment SM.lvclass">)  [unwired: 7 in]
        n347 = Bundle By Name(cluster=w643, "C.E."=w641) -> (w642:T30)
        n348 = call <vilib>:"Add State(s) to Queue__jki_lib_state_machine.vi"("State(s) in (\"\")"=w671) -> ("States Out"=w670:string)  [unwired: 14 in]
      }
      frame "---------- KH ----------" {
        n349 = call <vilib>:"Add State(s) to Queue__jki_lib_state_machine.vi"("State(s) in (\"\")"=w675) -> ("States Out"=w674:string)  [unwired: 14 in]
      }
      frame "KH: set KH 0" {
        # "initialize the Channel Settings array"
        # "remove duplicates"
        n350 = local read "KH Addresses"() -> (w688:refnum<visa-resource-name>[])
        n351 = call-poly <userlib>:"Remove Duplicates from 1D Array__ogtk.vi"("Input Array"=w688) -> ("Output Array"=w689:variant[])  [unwired: 1 out]
        n352 = Variant To Data(error in=w687, type=w688, Variant=w689) -> (data=w680:refnum<visa-resource-name>[], error out=w679:errorcluster)
        n353 = local write "KH Addresses"(w680) -> ()
        n354 = Initialize Array(T18 {"Channel"=enum."Channel 1", "Gain"=enum."10x", "Bandwidth Filter"=enum."ON", "Shunt Resistor"=enum."50 Ohms", "Coupling"=enum."DC", "Input Config"=enum."Differential"} ("Channel Settings"), 8 ("dimension size")) -> (w682:T18[])
        n355 = Bundle(w682) -> (w681:cluster{T18[]})  [unwired: 1 in]
        n356 = Array Size(array=w680) -> (size(s)=w685:i32)
        n357 = for {
          tunnel: w680 -> [_] mode=indexing
          tunnel: [w697] -> w676 mode=concatenating
          tunnel: w679 -> [w696]
          tunnel: [w695] -> w678
          i -> [w699]
          n358 = call "Number to Letter.vi"("Number"=w699) -> ("Letter"=w698:string)
          n359 = for {
            N: 8 -> [_]
            tunnel: w698 -> [w704]
            tunnel: [w703] -> w697 mode=indexing
            tunnel: w696 -> [w702]
            tunnel: [w701] -> w695
            i -> [w706]
            n360 = Increment(x=w706) -> (x+1=w700:i32)
            n361 = Format Into String(format string="%s %d", error in=w702, w704, w700) -> (resulting string=w703:string, error out=w701:errorcluster)  [unwired: 1 in]
          }
        }
        n362 = Initialize Array(w681, w685) -> (w686:cluster{T18[]}[])
        n363 = Bundle By Name(cluster=w691, "Channel Settings"=w686) -> (w690:T30)
        n364 = property on="Ring" class="Ring (strict)"(error in=w678, "Strings []"=w676) -> (error out=w677:errorcluster)  [unwired: 1 in, 1 out]
        n365 = call <vilib>:"Add State(s) to Queue__jki_lib_state_machine.vi"("State(s) in (\"\")"=w693) -> ("States Out"=w692:string)  [unwired: 14 in]
      }
      frame "KH: set KH 1" {
        n366 = Unbundle By Name(w718) -> ("Channel Settings"=w707:cluster{"Channel Setting":T27}[], "KH.KH #"=w720:u16[], "KH.KH Gain"=w723:T3[], "Lockin.Electrode Config"=w721:T6[], "KH.KH Shunt Resistor"=w722:T4[], "KH All Buttons"=w719:T8)
        n367 = local read "Bandwidth Filter"() -> (w708:bool)
        n368 = local read "DC Coupled"() -> (w709:bool)
        n369 = for {
          tunnel: w721 -> [w748] mode=indexing
          tunnel: w723 -> [w747] mode=indexing
          tunnel: w722 -> [w746] mode=indexing
          tunnel: w720 -> [w742] mode=indexing
          tunnel: [w751] -> w714 mode=indexing
          tunnel: w719 -> [w750]
          tunnel: [w749] -> w712 mode=indexing
          tunnel: [w745] -> w713 mode=indexing
          shift-right: [w738] -> w716
          shift-left: w707 -> [w739]
          tunnel: w709 -> [w734]
          tunnel: w708 -> [w729]
          n370 = property on="Ring" class="Ring (strict)"() -> ("Strings []"=w744:string[])  [unwired: 2 in, 2 out]
          n371 = case shown="\"No Selection\", Default" w750 {
            tunnel: w748 -> [w770 _ _]
            tunnel: [w775 Input_Configuration-Enum."Ground" ("Input Config") Input_Configuration-Enum."Differential" ("Input Config")] -> w745
            tunnel: w747 -> [w774 w793 w796]
            tunnel: [w773 w793 w796] -> w749
            tunnel: w746 -> [w772 _ _]
            tunnel: [w771 Shunt-Enum."Open" ("Shunt Resistor") w794] -> w751
            frame "No Selection", Default {
              n372 = case shown="\"Voltage (SE)\"" w770 {
                tunnel: [Input_Configuration-Enum."Ground" ("Input Config") Input_Configuration-Enum."Differential" ("Input Config") Input_Configuration-Enum."SE+ (-gnd)" ("Input Config") Input_Configuration-Enum."Differential" ("Input Config") Input_Configuration-Enum."Differential" ("Input Config")] -> w775
                tunnel: [Shunt-Enum."Open" ("Shunt Resistor") w779 Shunt-Enum."Open" ("Shunt Resistor") Shunt-Enum."Open" ("Shunt Resistor") Shunt-Enum."50k Ohms" ("Shunt Resistor")] -> w771
                tunnel: w774 -> [w776 w780 w783 w787 w789]
                tunnel: [w776 w780 w783 w787 w789] -> w773
                tunnel: w772 -> [_ w779 _ _ _]
                frame "Ground", Default {
                }
                frame "Current" {
                }
                frame "Voltage (SE)" {
                }
                frame "Voltage (Diff)" {
                }
                frame "Gate" {
                }
              }
            }
            frame "All Ground" {
            }
            frame "All Differential" {
              n373 = local read "Defualt Shunt Resistor"() -> (w794:T4)
            }
          }
          n374 = To Long Integer(number=w742) -> (32bit integer=w743:i32)
          n375 = Index Array(array=w744, index=w743) -> (element=w741:string)
          n376 = Select(t=Coupling-Enum."DC" ("Coupling"), s=w734, f=Coupling-Enum."AC" ("Coupling")) -> (s? t:f=w731:T21)
          n377 = Scan From String(format string="%s %d", input string=w741) -> (error out=w735:errorcluster, output 1=w737:string, output 2=w736:i32)  [unwired: 4 in, 2 out]
          n378 = Select(t=Filter-Enum."ON" ("Bandwidth Filter"), s=w729, f=Filter-Enum."OFF" ("Bandwidth Filter")) -> (s? t:f=w727:T20)
          n379 = case shown="No Error" w735 {
            tunnel: w751 -> [w768 _]
            tunnel: w749 -> [w767 _]
            tunnel: w745 -> [w766 _]
            tunnel: w739 -> [w758 w769]
            tunnel: [w757 w769] -> w738
            tunnel: w737 -> [w756 _]
            tunnel: w736 -> [w755 _]
            tunnel: w731 -> [w753 _]
            tunnel: w727 -> [w752 _]
            frame No Error {
              n380 = Decrement(x=w755) -> (x-1=w754:i32)
              n381 = call "Letter to Number.vi"("Letter"=w756) -> ("Number"=w759:i32)
              n382 = Index Array(array=w758, index=w759) -> (element=w764:cluster{"Channel Setting":T27})
              n383 = Unbundle(w764) -> ("Channel Setting"=w763:T27)
              n384 = Index Array(array=w763, index=w754) -> (element=w762:T18)
              n385 = Bundle By Name(cluster=w762, "Channel"=w754, "Gain"=w767, "Input Config"=w766, "Shunt Resistor"=w768, "Coupling"=w753, "Bandwidth Filter"=w752) -> (w761:T18)
              n386 = Replace Array Subset(array=w763, new element=w761, index=w754) -> (w765:T27)
              n387 = Bundle("Channel Setting"=w765) -> (w760:cluster{"Channel Setting":T27})  [unwired: 1 in]
              n388 = Replace Array Subset(array=w758, new element=w760, index=w759) -> (w757:cluster{"Channel Setting":T27}[])
            }
            frame Error {
            }
          }
        }
        n389 = Bundle By Name(cluster=w718, "Channel Settings"=w716, "KH.KH Gain"=w712, "KH.KH Configuration"=w713, "KH.KH Shunt Resistor"=w714) -> (w724:T30)
        n390 = local write "KH All Buttons"(T8."No Selection" ("KH All Buttons")) -> ()
        n391 = local read "KH"() -> (w715:T5)
        n392 = Bundle By Name(cluster=w715, "KH Gain"=w712, "KH Configuration"=w713, "KH Shunt Resistor"=w714) -> (w711:T5)
        n393 = local write "KH"(w711) -> ()
        n394 = call <vilib>:"Add State(s) to Queue__jki_lib_state_machine.vi"("State(s) in (\"\")"=w726) -> ("States Out"=w725:string)  [unwired: 14 in]
      }
      frame "KH: set KH 2" {
        n395 = Unbundle By Name(w804) -> ("Channel Settings"=w809:cluster{"Channel Setting":T27}[])
        n396 = Unbundle By Name(w804) -> ("C.E."=w801:refnum<class "Control Experiment SM.lvclass">)
        n397 = Unbundle By Name(w801) -> ("KH7008"=w800:refnum<class "Instrument.KH7008.lvclass">[])
        n398 = for {
          tunnel: w799 -> [w824]
          tunnel: [w816] -> w797
          tunnel: w809 -> [w823] mode=indexing
          tunnel: w800 -> [w822] mode=indexing
          tunnel: [w815] -> w805 mode=concatenating
          tunnel: [w814] -> w798 mode=indexing
          n399 = Unbundle(w823) -> ("Channel Setting"=w819:T27)
          n400 = call <userlib>:"Write Channel Setting.vi"("error in (no error)"=w824, "Channel Setting"=w819, "KH7008 in"=w822) -> ("error out"=w820:errorcluster, "KH7008 out"=w821:refnum<class "Instrument.KH7008.lvclass">)  [unwired: 7 in]
          n401 = call <userlib>:"KH Control.vi"("error in"=w820, "KH7008.lvclass"=w821) -> ("error out"=w818:errorcluster, "KH7008.lvclass out"=w817:refnum<class "Instrument.KH7008.lvclass">)  [unwired: 8 in]
          n402 = call <userlib>:"Read Gain.vi"("error in (no error)"=w818, "KH7008 in"=w817) -> ("error out"=w816:errorcluster, "Gain"=w815:dbl[], "KH7008 out"=w814:refnum<class "Instrument.KH7008.lvclass">)  [unwired: 7 in]
        }
        n403 = local read "Gain"() -> (w806:dbl[])
        n404 = Bundle By Name(cluster=w801, "KH7008"=w798) -> (w803:refnum<class "Control Experiment SM.lvclass">)
        n405 = call "Multiply Gains.vi"("Other Gain"=w806, "Gain"=w805) -> ("Gain x Other Gain"=w808:dbl[])
        n406 = Unbundle By Name(w803) -> ("Lockin"=w802:refnum<class "Instrument.Lockin.lvclass">)
        n407 = call <userlib>:"setGain.vi"("error in (no error)"=w797, "Gain"=w808, "Instrument.Lockin in"=w802) -> ("error out"=w807:errorcluster)  [unwired: 7 in, 1 out]
        n408 = Bundle By Name(cluster=w804, "C.E."=w803) -> (w811:T30)
        n409 = call <vilib>:"Clear Errors.vi"("error in (no error)"=w807) -> ("error out"=w810:errorcluster)  [unwired: 5 in, 1 out]
        n410 = call <vilib>:"Add State(s) to Queue__jki_lib_state_machine.vi"("State(s) in (\"\")"=w813) -> ("States Out"=w812:string)  [unwired: 14 in]
      }
      frame "---------- Instruments ----------" {
        n411 = call <vilib>:"Add State(s) to Queue__jki_lib_state_machine.vi"("State(s) in (\"\")"=w828) -> ("States Out"=w827:string)  [unwired: 14 in]
      }
      frame "Instruments: Load Classes" {
        n412 = Unbundle By Name(w834) -> ("C.E."=w832:refnum<class "Control Experiment SM.lvclass">)
        n413 = call "Load Instrument Classes.vi"("error in (no error)"=w829, "Control Experiment.lvclass"=w832) -> ("error out"=w830:errorcluster, "Control Experiment out"=w831:refnum<class "Control Experiment SM.lvclass">)  [unwired: 8 in]
        n414 = Bundle By Name(cluster=w834, "C.E."=w831) -> (w833:T30)
        n415 = call <vilib>:"Add State(s) to Queue__jki_lib_state_machine.vi"("State(s) in (\"\")"=w836) -> ("States Out"=w835:string)  [unwired: 14 in]
      }
      frame "Instruments: Initialize KH" {
        n416 = Unbundle By Name(w840) -> ("C.E."=w841:refnum<class "Control Experiment SM.lvclass">)
        n417 = Unbundle By Name(w841) -> ("KH7008"=w843:refnum<class "Instrument.KH7008.lvclass">[])
        n418 = for {
          tunnel: w843 -> [w849]
          tunnel: [w853] -> w837 mode=indexing
          tunnel: w845 -> [w852]
          tunnel: [w851] -> w844
          tunnel: "KH Addresses" -> [w850] mode=indexing
          n419 = Index Array(array=w849) -> (element=w848:refnum<class "Instrument.KH7008.lvclass">)  [unwired: 1 in]
          n420 = call-dynamic "Open.vi"("error in (no error)"=w852, "Address"=w850, "Instrument.KH7008 in"=w848) -> ("error out"=w851:errorcluster, "Instrument.KH7008 out"=w853:refnum<class "Instrument.KH7008.lvclass">)  [unwired: 7 in]
        }
        n421 = Bundle By Name(cluster=w841, "KH7008"=w837) -> (w838:refnum<class "Control Experiment SM.lvclass">)
        n422 = Bundle By Name(cluster=w840, "C.E."=w838) -> (w839:T30)
        n423 = call <vilib>:"Add State(s) to Queue__jki_lib_state_machine.vi"("State(s) in (\"\")"=w847) -> ("States Out"=w846:string)  [unwired: 14 in]
      }
      frame "Instruments: Initialize Lockin" {
        n424 = Unbundle By Name(w860) -> ("C.E."=w856:refnum<class "Control Experiment SM.lvclass">)
        n425 = Unbundle By Name(w856) -> ("Lockin"=w857:refnum<class "Instrument.Lockin.lvclass">)
        n426 = call-dynamic "Open.vi"("error in (no error)"=w861, "Address"="Lockin Address", "Instrument.Lockin in"=w857) -> ("error out"=w858:errorcluster, "Instrument.Lockin out"=w855:refnum<class "Instrument.Lockin.lvclass">)  [unwired: 7 in]
        n427 = Bundle By Name(cluster=w856, "Lockin"=w855) -> (w854:refnum<class "Control Experiment SM.lvclass">)
        n428 = Bundle By Name(cluster=w860, "C.E."=w854) -> (w859:T30)
        n429 = call <vilib>:"Add State(s) to Queue__jki_lib_state_machine.vi"("State(s) in (\"\")"=w864) -> ("States Out"=w863:string)  [unwired: 14 in]
      }
      frame "Instruments: Initialize Instruments" {
        n430 = Unbundle By Name(w871) -> ("C.E."=w870:refnum<class "Control Experiment SM.lvclass">)
        n431 = Unbundle By Name(w870) -> ("Capacitance Bridge"=w876:refnum<class "Instrument.CBridge.lvclass">, "Strain Cell"=w866:refnum<class "Instrument.Strain.lvclass">)
        n432 = call-dynamic "Open.vi"("error in (no error)"=w872, "Address"="Capacitance Bridge Address", "Instrument in"=w876) -> ("error out"=w875:errorcluster, "Instrument out"=w869:refnum<class "Instrument.CBridge.lvclass">)  [unwired: 7 in]
        n433 = call-dynamic "Open.vi"("error in (no error)"=w875, "Address"="Strain Cell Address", "Instrument in"=w866) -> ("error out"=w865:errorcluster, "Instrument out"=w867:refnum<class "Instrument.Strain.lvclass">)  [unwired: 7 in]
        n434 = Bundle By Name(cluster=w870, "Capacitance Bridge"=w869, "Strain Cell"=w867) -> (w868:refnum<class "Control Experiment SM.lvclass">)
        n435 = Bundle By Name(cluster=w871, "C.E."=w868) -> (w877:T30)
        n436 = call <vilib>:"Add State(s) to Queue__jki_lib_state_machine.vi"("State(s) in (\"\")"=w879) -> ("States Out"=w878:string)  [unwired: 14 in]
      }
      frame "---------- Asana ----------" {
        n437 = call <vilib>:"Add State(s) to Queue__jki_lib_state_machine.vi"("State(s) in (\"\")"=w883) -> ("States Out"=w882:string)  [unwired: 14 in]
      }
      frame "Asana: Initialize Authentication Info" {
        n438 = Bundle By Name(cluster=w885, "Asana.Authentication Info.Client ID"="1150712142949183" ("Client ID"), "Asana.Authentication Info.Client Secret"="530770942aed47201cd52aeb331bdd57" ("Client Secret"), "Asana.Authentication Info.Redirect URI"="https://www.google.com/" ("Redirect URI")) -> (w884:T30)
        n439 = call <vilib>:"Add State(s) to Queue__jki_lib_state_machine.vi"("State(s) in (\"\")"=w891) -> ("States Out"=w890:string)  [unwired: 14 in]
      }
      frame "Asana: Authenticate" {
        n440 = Unbundle By Name(w893) -> ("Asana.Time Stamp"=w907:timestamp, "Asana.Refresh Token"=w894:string, "Asana.Authentication Info"=w897:T36)
        n441 = Get Date/Time In Seconds() -> (seconds since 1Jan1904=w906:timestamp)
        n442 = Subtract(x=w907, y=w906) -> (x-y=w905:dbl)
        n443 = Less?(x=w905, y=3600.0) -> (x < y?=w898:bool)
        n444 = Select(t=w894, s=w898, f="" ("t")) -> (s? t:f=w896:string)
        n445 = call <userlib>:"Asana Authentication.vi"("error in (no error)"=w892, "Authentication Info"=w897, "Refresh Token In"=w896) -> ("error out"=w901:errorcluster, "Authentication Header"=w900:T29[], "Refresh Token Out"=w899:string)  [unwired: 5 in, 1 out]
        n446 = case shown="No Error" w901 {
          selector: w901 -> [w911 _]
          tunnel: w900 -> [w912 _]
          tunnel: w899 -> [w910 _]
          tunnel: w893 -> [w915 w917]
          tunnel: [w913 w917] -> w903
          tunnel: [w911 errorcluster {"status"=FALSE, "code"=0, "source"=""} ("error in (no error)")] -> w902
          frame No Error {
            n447 = Get Date/Time In Seconds() -> (seconds since 1Jan1904=w914:timestamp)
            n448 = Bundle By Name(cluster=w915, "Asana.Refresh Token"=w910, "Asana.Authentication Header"=w912, "Asana.Time Stamp"=w914) -> (w913:T30)
            "Refresh Token Out" <- w910
          }
          frame Error {
          }
        }
        n449 = call <vilib>:"Add State(s) to Queue__jki_lib_state_machine.vi"("State(s) in (\"\")"=w909) -> ("States Out"=w908:string)  [unwired: 14 in]
      }
      frame "Asana: Get Teams and Projects" {
        # "task"
        # "project"
        # "team"
        n450 = Unbundle By Name(w925) -> ("Asana.Authentication Header"=w921:T29[])
        n451 = Unbundle By Name(w925) -> ("Experiment.Device"=w918:string)
        n452 = call <userlib>:"Get Teams.vi"("Authorization"=w921, "error in (no error)"=w938) -> ("error out"=w937:errorcluster, "Teams Out"=w927:T37)  [unwired: 8 in]
        n453 = Format Into String(error in=w937, T22."Samples" ("Team")) -> (resulting string=w936:string, error out=w935:errorcluster)  [unwired: 2 in]
        n454 = call "Asana Dictionary Get Value.vi"("error in (no error)"=w935, "Key"=w936, "Data"=w927) -> ("error out"=w932:errorcluster, "Value"=w934:string)  [unwired: 7 in]
        n455 = call <userlib>:"Get Projects.vi"("Authorization"=w921, "error in (no error)"=w932, "Team GID"=w934) -> ("error out"=w931:errorcluster, "Projects Out"=w929:T37)  [unwired: 7 in]
        n456 = call "Asana Dictionary Get Value.vi"("error in (no error)"=w931, "Key"="Devices" ("element"), "Data"=w929) -> ("error out"=w930:errorcluster, "Value"=w919:string)  [unwired: 7 in]
        n457 = call <userlib>:"Get Tasks.vi"("Authorization"=w921, "error in (no error)"=w930, "Project GID"=w919) -> ("error out"=w926:errorcluster, "data"=w928:T38)  [unwired: 7 in]
        n458 = call "Asana Dictionary Tasks Get Value.vi"("error in (no error)"=w926, "Key"=w918, "data"=w928) -> ("error out"=w923:errorcluster, "Value"=w924:string)  [unwired: 7 in]
        n459 = case shown="\"\"" w924 {
          tunnel: w923 -> [w941 w946]
          tunnel: [w941 w945] -> w922
          tunnel: w921 -> [_ w944]
          tunnel: w919 -> [_ w943]
          tunnel: w918 -> [_ w942]
          frame Default {
          }
          frame "" {
            # "empty means\ntask doesn't\nexist"
            n460 = case shown="Default" w942 {
              selector: w942 -> [_ w948]
              tunnel: w946 -> [w947 w952]
              tunnel: [w947 w951] -> w945
              tunnel: w944 -> [_ w950]
              tunnel: w943 -> [_ w949]
              frame "" {
              }
              frame Default {
                n461 = call <userlib>:"Create Task.vi"("Authorization"=w950, "error in (no error)"=w952, "Name"=w948, "Project GID"=w949) -> ("error out"=w951:errorcluster)  [unwired: 6 in, 1 out]
              }
            }
          }
        }
        n462 = call <vilib>:"Add State(s) to Queue__jki_lib_state_machine.vi"("State(s) in (\"\")"=w940) -> ("States Out"=w939:string)  [unwired: 14 in]
      }
      frame "---------- Experiment VI ----------" {
        n463 = call <vilib>:"Add State(s) to Queue__jki_lib_state_machine.vi"("State(s) in (\"\")"=w956) -> ("States Out"=w955:string)  [unwired: 14 in]
      }
      frame "Experiment VI: Populate VI Ring" {
        n464 = call <userlib>:"Current VIs Parent Directory__ogtk.vi"() -> ("Parent Directory (+ Relative)"=w973:path)  [unwired: 5 in]
        n465 = call <userlib>:"String to 1D Array__ogtk.vi"("delimiter (Tab)"="\n", "string"="----Sweep Control----\nSweep Control.vi\nContinuous B Sweep.vi") -> ("Array of Strings"=w959:string[])  [unwired: 9 in]
        n466 = call <userlib>:"String to 1D Array__ogtk.vi"("delimiter (Tab)"="\n", "string"="----Transport----\nIV.vi\nIV_Sweep.vi\nLockin_time.vi\nLockin_Vsg.vi\nLockin_sweep.vi\nLockin_AIWFM_time.vi\nTHz_TimeDelay.vi\nSweep_AIWFM_time.vi") -> ("Array of Strings"=w958:string[])  [unwired: 9 in]
        n467 = Strip Path(path=w973) -> (stripped path=w970:path)  [unwired: 1 out]
        n468 = Build Path(base path=w970, name or relative path="SweepControl") -> (appended path=w969:path)
        n469 = Build Path(base path=w970, name or relative path="Transport") -> (appended path=w965:path)
        n470 = for {
          tunnel: w969 -> [w983]
          tunnel: w959 -> [w982] mode=indexing
          tunnel: [w981] -> w962 mode=indexing
          n471 = Build Path(base path=w983, name or relative path=w982) -> (appended path=w981:path)
        }
        n472 = for {
          tunnel: w965 -> [w980]
          tunnel: w958 -> [w979] mode=indexing
          tunnel: [w978] -> w961 mode=indexing
          n473 = Build Path(base path=w980, name or relative path=w979) -> (appended path=w978:path)
        }
        n474 = Build Array (concatenate)(w962, w961) -> (w960:path[])
        n475 = Build Array (concatenate)(w959, w958) -> (w957:string[])
        n476 = Bundle By Name(cluster=w964, "VI paths"=w960) -> (w963:T30)
        n477 = property on="Ring" class="Ring (strict)"("Strings []"=w957) -> ()  [unwired: 2 in, 2 out]
        n478 = call <vilib>:"Add State(s) to Queue__jki_lib_state_machine.vi"("State(s) in (\"\")"=w977) -> ("States Out"=w976:string)  [unwired: 14 in]
      }
      frame "Experiment VI: Open VI" {
        n479 = Unbundle By Name(w989) -> ("VI paths"=w988:path[])
        n480 = Index Array(array=w988, index="Ring") -> (element=w986:path)
        n481 = call "Open Experiment VI.vi"("error in (no error)"=w985, "Path"=w986) -> ("error out"=w984:errorcluster)  [unwired: 9 in]
        n482 = call <vilib>:"Add State(s) to Queue__jki_lib_state_machine.vi"("State(s) in (\"\")"=w991) -> ("States Out"=w990:string)  [unwired: 14 in]
      }
      frame "Experiment VI: Open Lockin" {
        n483 = call "Open Lockin.vi"("error in (no error)"=w993) -> ("error out"=w992:errorcluster)  [unwired: 10 in]
        n484 = call <vilib>:"Add State(s) to Queue__jki_lib_state_machine.vi"("State(s) in (\"\")"=w996) -> ("States Out"=w995:string)  [unwired: 14 in]
      }
      frame "---------- PGSQL ----------" {
        n485 = call <vilib>:"Add State(s) to Queue__jki_lib_state_machine.vi"("State(s) in (\"\")"=w1000) -> ("States Out"=w999:string)  [unwired: 14 in]
      }
      frame "PGSQL: Start Logger" {
        n486 = Unbundle By Name(w1002) -> ("Logger"=w1007:refnum<class "Logger.PGSQL.lvclass">)
        n487 = call <vilib>:"Create.vi"("error in (no error)"=w1004, "SMO"=w1007) -> ("error out"=w1006:errorcluster, "SMO out"=w1008:refnum<class "Logger.PGSQL.lvclass">)  [unwired: 7 in, 1 out]
        n488 = call <vilib>:"Start.vi"("error in (no error)"=w1006, "SMO"=w1008) -> ("error out"=w1003:errorcluster, "SMO out"=w1005:refnum<class "Logger.PGSQL.lvclass">)  [unwired: 8 in]
        n489 = Bundle By Name(cluster=w1002, "Logger"=w1005) -> (w1001:T30)
        n490 = call <vilib>:"Add State(s) to Queue__jki_lib_state_machine.vi"("State(s) in (\"\")"=w1010) -> ("States Out"=w1009:string)  [unwired: 14 in]
      }
      frame "PGSQL: Write" {
        w1022 = "" ("f")
        n491 = Unbundle By Name(w1026) -> ("Logger"=w1020:refnum<class "Logger.PGSQL.lvclass">, "Experiment.Instrument"=w1011:T9, "Experiment.Device"=w1025:string, "Experiment.User"=w1024:string)
        n492 = local read "I'm Finished Taking Data!"() -> (w1023:bool)
        n493 = Not(x=w1023) -> (.not. x?=w1021:bool)
        n494 = call "Device and User PGSQL Paths.vi"("instrument"=w1011) -> ("User Path"=w1013:string, "Device Path"=w1019:string)  [unwired: 5 in]
        n495 = Select(t=w1025, s=w1021, f=w1022) -> (s? t:f=w1018:string)
        n496 = Select(t=w1024, s=w1021, f=w1022) -> (s? t:f=w1012:string)
        n497 = call <userlib>:"Logger.PGSQL.WriteVariable.vi"("error in (no error)"=w1016, "Data"=w1018, "Address"=w1019, "Logger"=w1020) -> ("error out"=w1015:errorcluster, "Logger out"=w1017:refnum<class "Logger.PGSQL.lvclass">)  [unwired: 6 in]
        n498 = call <userlib>:"Logger.PGSQL.WriteVariable.vi"("error in (no error)"=w1015, "Data"=w1012, "Address"=w1013, "Logger"=w1017) -> ("error out"=w1014:errorcluster)  [unwired: 6 in, 1 out]
        n499 = call <vilib>:"Add State(s) to Queue__jki_lib_state_machine.vi"("State(s) in (\"\")"=w1028) -> ("States Out"=w1027:string)  [unwired: 14 in]
      }
      frame "---------- Pickering ----------" {
        n500 = call <vilib>:"Add State(s) to Queue__jki_lib_state_machine.vi"("State(s) in (\"\")"=w1032) -> ("States Out"=w1031:string)  [unwired: 14 in]
      }
      frame "Pickering: Pickering config" {
        n501 = Unbundle By Name(w1034) -> ("C.E."=w1033:refnum<class "Control Experiment SM.lvclass">)
        n502 = case shown="\"Write\", Default" w1037 {
          tunnel: w1035 -> [w1049 w1054]
          tunnel: [w1048 w1053] -> w1036
          tunnel: w1033 -> [w1047 w1055]
          frame "Write", Default {
            n503 = Bundle("Electrodes (Pickering)"="Electrodes (Pickering)", "X Channels"="X Channels") -> (w1041:T39)  [unwired: 1 in]
            n504 = Bundle("Labels (Pickering)"="Labels (Pickering)", "Y Channels"="Y Channels") -> (w1040:T40)  [unwired: 1 in]
            n505 = Bundle(w1041, w1040) -> (w1046:T41)  [unwired: 1 in]
            n506 = call "PickeringWriteConfig Asynchronous.vi"("error in (no error)"=w1049, "Pickering Config"=w1046, "Control Experiment in"=w1047) -> ("error out"=w1048:errorcluster)  [unwired: 7 in, 1 out]
          }
          frame "Read" {
            n507 = call "PickeringReadConfig Asynchronous.vi"("error in (no error)"=w1054, "Control Experiment in"=w1055) -> ("error out"=w1053:errorcluster, "Pickering Config"=w1052:T42)  [unwired: 7 in, 1 out]
            n508 = Unbundle By Name(w1052) -> ("x config.Electrode"=w1057:T12, "x config.X Channels"=w1051:string[], "y config.Label"=w1056:u16[], "y config.Y Channels"=w1050:string[][])
            n509 = local write "Electrodes (Pickering)"(w1057) -> ()
            n510 = local write "Labels (Pickering)"(w1056) -> ()
            n511 = local write "X Channels"(w1051) -> ()
            n512 = local write "Y Channels"(w1050) -> ()
          }
        }
        n513 = call <vilib>:"Add State(s) to Queue__jki_lib_state_machine.vi"("State(s) in (\"\")"=w1039) -> ("States Out"=w1038:string)  [unwired: 14 in]
      }
      frame "Pickering: set Pickering" {
        n514 = local read "Electrodes (Pickering)"() -> (w1068:T12)
        n515 = local read "Labels (Pickering)"() -> (w1065:u16[])
        n516 = Unbundle By Name(w1060) -> ("C.E."=w1059:refnum<class "Control Experiment SM.lvclass">)
        n517 = call "ElectrodesLabelsToPickeringChannels.vi"("error in (no error)"=w1064, "Labels"=w1065, "Electrodes"=w1068, "Control Experiment in"=w1059) -> ("error out"=w1067:errorcluster, "Y Channel Array"=w1061:string[][], "X Channel Array"=w1062:string[], "Control Experiment out"=w1058:refnum<class "Control Experiment SM.lvclass">)  [unwired: 4 in]
        "X Channel Array" <- w1062
        "Y Channel Array" <- w1061
        n518 = case shown="\"Pickering 4 Wire PPMS DR\"" "Pickering Enum" {
          tunnel: w1067 -> [w1075 w1089]
          tunnel: [w1074 w1088] -> w1066
          tunnel: w1062 -> [w1072 _]
          tunnel: w1061 -> [w1073 w1076]
          tunnel: w1058 -> [w1071 w1087]
          frame "Pickering 4 Wire", Default {
            n519 = call "Pickering 4 Wire Asynchronous.vi"("error in (no error)"=w1075, "Y Channel Array"=w1073, "X Channel Array"=w1072, "Control Experiment in"=w1071) -> ("error out"=w1074:errorcluster)  [unwired: 6 in, 1 out]
          }
          frame "Pickering 4 Wire PPMS DR" {
            n520 = Index Array(array=w1076) -> (element #1=w1085:string[], element #2=w1084:string[], element #3=w1083:string[], element #4=w1082:string[], element #5=w1081:string[], element #6=w1080:string[], element #7=w1079:string[], element #8=w1078:string[])  [unwired: 16 in]
            n521 = Bundle(cluster=T23 {"26"=[], "27"=[], "28"=[], "1"=[], "2"=[], "3"=[], "4"=[], "5"=[]} ("Channel Cluster"), "26"=w1085, "27"=w1084, "28"=w1083, "1"=w1082, "2"=w1081, "3"=w1080, "4"=w1079, "5"=w1078) -> (w1077:T23)
            n522 = call "Pickering 4 Wire PPMS DR Asynchronous.vi"("error in (no error)"=w1089, "Channel Cluster"=w1077, "Control Experiment in"=w1087) -> ("error out"=w1088:errorcluster)  [unwired: 7 in, 1 out]
          }
        }
        n523 = call <vilib>:"Add State(s) to Queue__jki_lib_state_machine.vi"("State(s) in (\"\")"=w1070) -> ("States Out"=w1069:string)  [unwired: 14 in]
      }
    }
  }
  n524 = Unbundle By Name(w2) -> ("C.E."=→"Control Experiment":refnum<class "Control Experiment SM.lvclass">)
